vi "Dielectric vs Temperature - freq (4192A) Delay - Copy.vi"() -> ()   [LabVIEW 2013]
uses:
  <vilib>/Instr/_visa.llb/VISA Configure Serial Port (Instr).vi
  <vilib>/Utility/file.llb/Write To Spreadsheet File (DBL).vi
  Instance           5 32Saved   K vs Temp - freq (4284A) .vi
  Instance           6 32Saved   K vs Temp - freq (4284A) .vi
  Instance          15 32Saved   K vs Temp - freq (4284A) .vi
  Instance          16 32Saved   K vs Temp - freq (4284A) .vi
  Instance           7 32Saved   K vs Temp - freq (4284A) .vi
  Instance           8 32Saved   K vs Temp - freq (4284A) .vi
  Instance           9 32Saved   K vs Temp - freq (4284A) .vi
  Instance          10 32Saved   K vs Temp - freq (4284A) .vi
  Instance          11 32Saved   K vs Temp - freq (4284A) .vi
  Instance          12 32Saved   K vs Temp - freq (4284A) .vi
  Instance          13 32Saved   K vs Temp - freq (4284A) .vi
  Instance          14 32Saved   K vs Temp - freq (4284A) .vi
  Instance          17 32Saved   K vs Temp - freq (4284A) .vi
  Instance          18 32Saved   K vs Temp - freq (4284A) .vi
  Instance          19 32Saved   K vs Temp - freq (4284A) .vi
  Instance          20 32Saved   K vs Temp - freq (4284A) .vi
  Instance          21 32Saved   K vs Temp - freq (4284A) .vi
  Instance          22 32Saved   K vs Temp - freq (4284A) .vi
  Instance          23 32Saved   K vs Temp - freq (4284A) .vi
  Instance          25 32Saved   K vs Temp - freq (4284A) .vi
  Instance          24 32Saved   K vs Temp - freq (4284A) .vi
  Instance          26 32Saved   K vs Temp - freq (4284A) .vi
panel:
  in  "Freq Value (Hz) (1MHz)":dbl=1000000.0
  out "tand1M":dbl
  out "K1M":dbl
  out "C1M":dbl
  out "Temp1MHz":dbl format="%#_3g"
  in  "Freq Value (Hz) (500kHz)":dbl=500000.0
  out "tand500k":dbl
  out "K500k":dbl
  out "C500k":dbl
  out "Temp500kHz":dbl format="%#_3g"
  in  "Freq Value (Hz) (250kHz)":dbl=250000.0
  out "tand250k":dbl
  out "K250k":dbl
  out "C250k":dbl
  out "Temp250kHz":dbl format="%#_3g"
  in  "Freq Value (Hz) (100kHz)":dbl=100000.0
  out "tand100k":dbl
  out "K100k":dbl
  out "C100k":dbl
  out "Temp100kHz":dbl format="%#_3g"
  in  "Freq Value (Hz) (50kHz)":dbl=50000.0
  out "tand50k":dbl
  out "K50k":dbl
  out "C50k":dbl
  out "Temp50kHz":dbl format="%#_3g"
  in  "Freq Value (Hz) (25kHz)":dbl=25000.0
  out "tand25k":dbl
  out "K25k":dbl
  out "C25k":dbl
  out "Temp25kHz":dbl format="%#_3g"
  in  "Freq Value (Hz) (10kHz)":dbl=10000.0
  out "tand10k":dbl
  out "K10k":dbl
  out "C10k":dbl
  out "Temp10kHz":dbl format="%#_3g"
  in  "Freq Value (Hz) (5kHz)":dbl=5000.0
  out "tand5k":dbl
  out "K5k":dbl
  out "C5k":dbl
  out "Temp5kHz":dbl format="%#_3g"
  in  "Freq Value (Hz) (2.5kHz)":dbl=2500.0
  out "tand2.5k":dbl
  out "K2.5k":dbl
  out "C2.5k":dbl
  out "Temp2.5kHz":dbl format="%#_3g"
  in  "Freq Value (Hz) (1kHz)":dbl=1000.0
  out "tand1k":dbl
  out "K1k":dbl
  out "C1k":dbl
  out "Temp1kHz":dbl format="%#_3g"
  in  "tand500k":dbl[](array[numeric])
  in  "K500k":dbl[](array[numeric])
  in  "Temp500k":dbl[](array[numeric])
  out "Temp500Hz":dbl format="%#_3g"
  out "C500":dbl
  out "?":dbl
  out "tand500":dbl
  in  "Freq Value (Hz) (500Hz)":dbl=500.0
  in  "Freq Value (Hz) (250Hz)":dbl=250.0
  in  "Freq Value (Hz) (100Hz)":dbl=100.0
  in  "Freq Value (Hz) (50Hz)":dbl=50.0
  in  "Freq Value (Hz) (25Hz)":dbl=25.0
  in  "tand100k":dbl[](array[numeric])
  in  "tand10k":dbl[](array[numeric])
  in  "tand1k":dbl[](array[numeric])
  in  "tand100":dbl[](array[numeric])
  in  "K100k":dbl[](array[numeric])
  in  "K10k":dbl[](array[numeric])
  in  "K1k":dbl[](array[numeric])
  in  "K100":dbl[](array[numeric])
  in  "Temp100k":dbl[](array[numeric])
  in  "Temp10k":dbl[](array[numeric])
  in  "Temp1k":dbl[](array[numeric])
  in  "Temp100":dbl[](array[numeric])
  out "Temp250Hz":dbl format="%#_3g"
  out "Temp100Hz":dbl format="%#_3g"
  out "tand25":dbl
  out "Temp50Hz":dbl format="%#_3g"
  in  "Start":bool
  out "Thickness":dbl
  out "Area":dbl
  in  "stop":bool
  out "tand250":dbl
  out "tand100":dbl
  out "tand50":dbl
  out "K250":dbl
  out "K100":dbl
  out "K50":dbl
  out "K25":dbl
  out "C250":dbl
  out "C100":dbl
  out "C50":dbl
  out "C25":dbl
  out "Temp25Hz":dbl format="%#_3g"
  out "Dielectric Loss vs. Temperature":cluster{"Y":dbl[], "Y":dbl[]}[](graph)
  out "Relative Permittivity vs. Temperature":cluster{"Y":dbl[], "Y":dbl[]}[](graph)
  in  "Comment (Sample's Name, compositions, whatever you want,..)":string
  in  "Thickness (mm)":dbl
  in  "Diameter (mm)":dbl
  in  "Path & File Name (*.txt)":path
  # "Temperature (C)"
  # "Frequency (Hz)"
  # "Capacitance (F)"
  # "Relative Permittivity"
  # "Dielectric Loss"
  # "Sample Details"
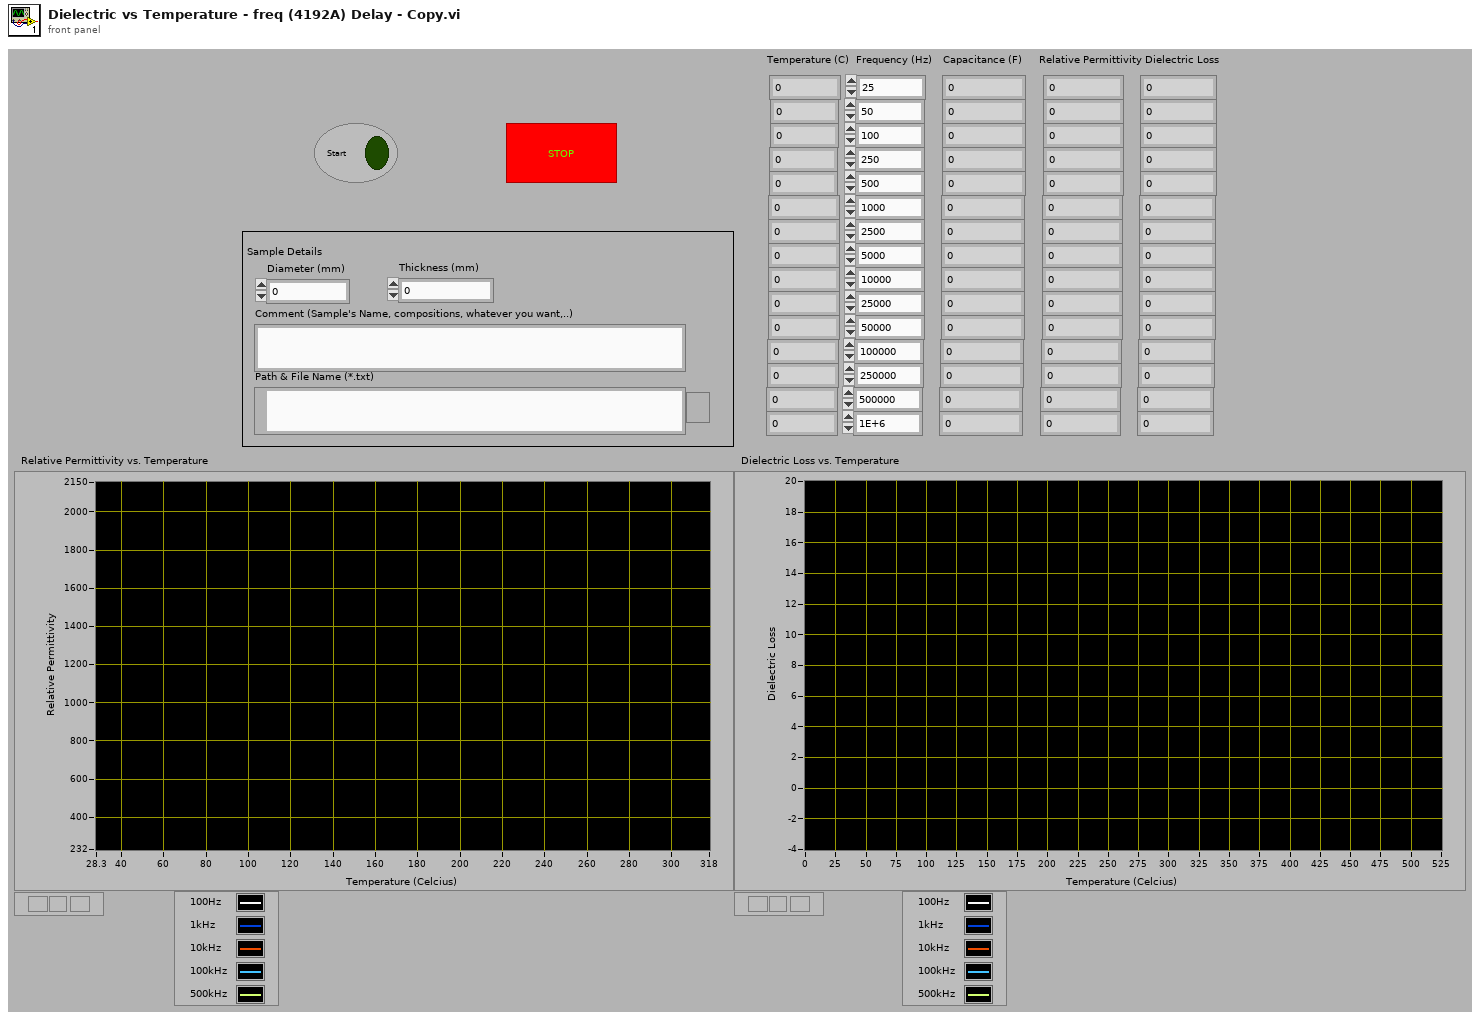
[diagram p1: front panel]
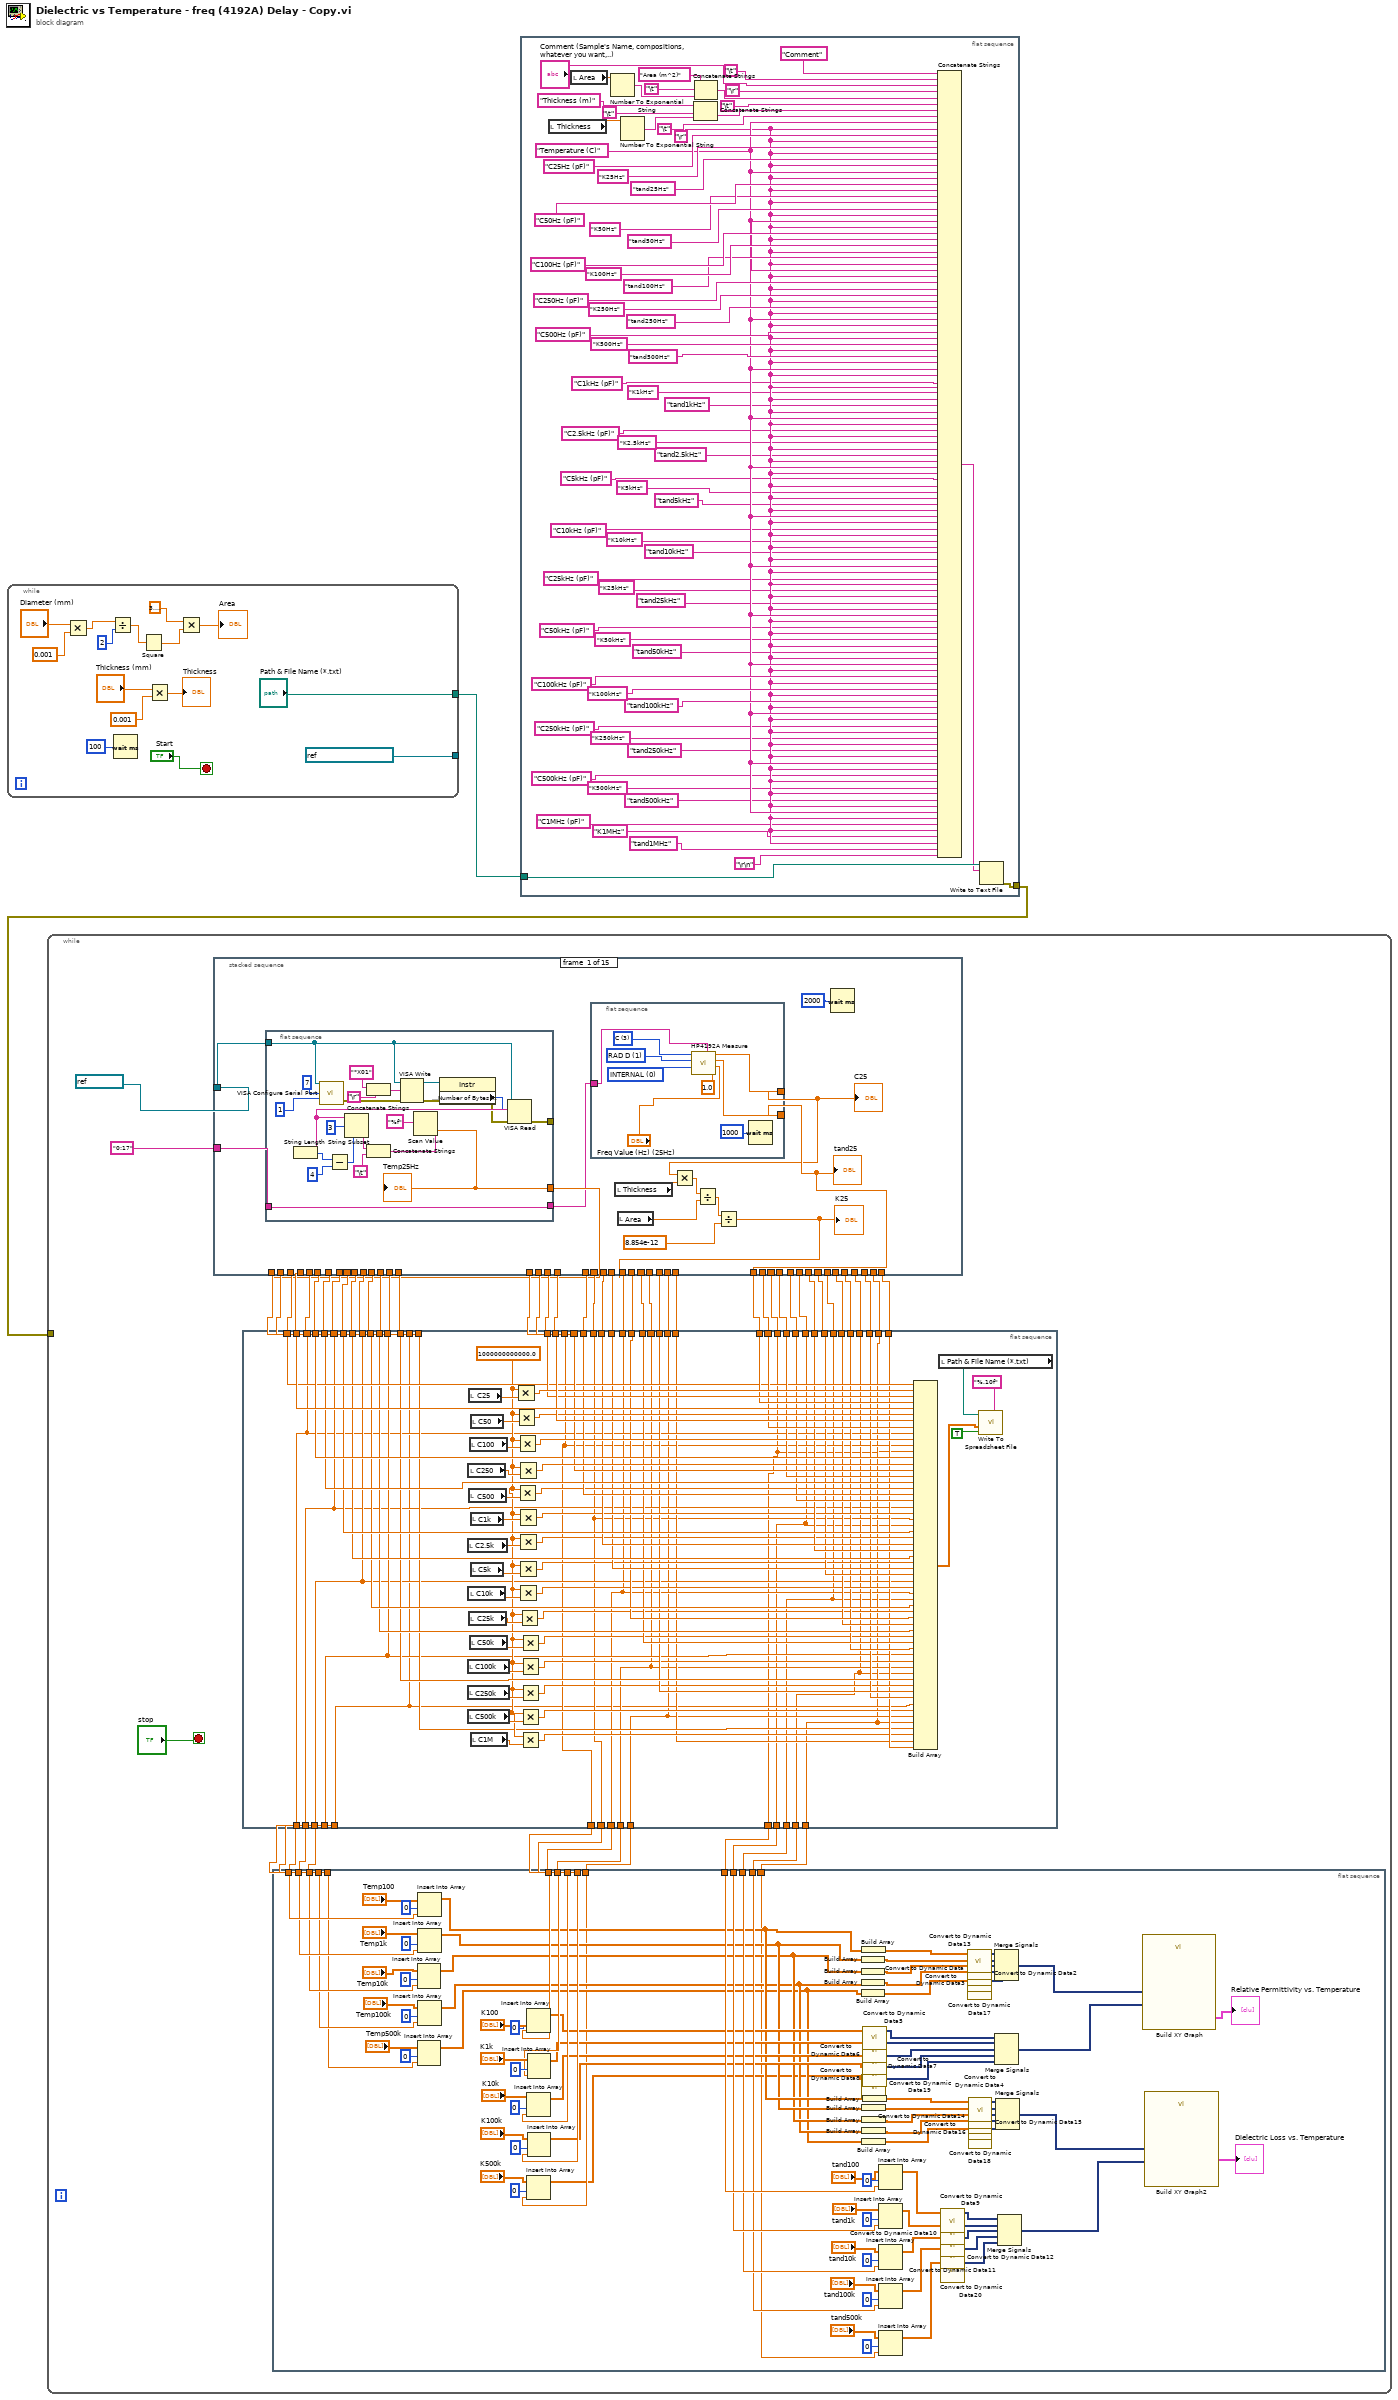
[diagram p0: block diagram]
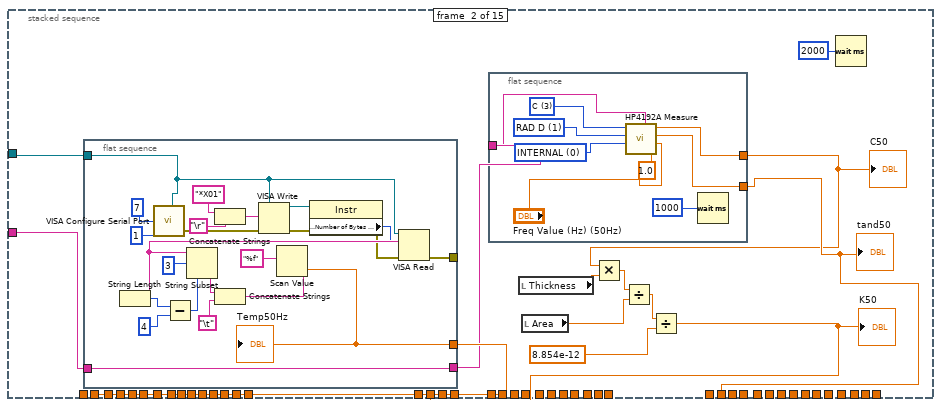
[diagram p2: hidden frame]
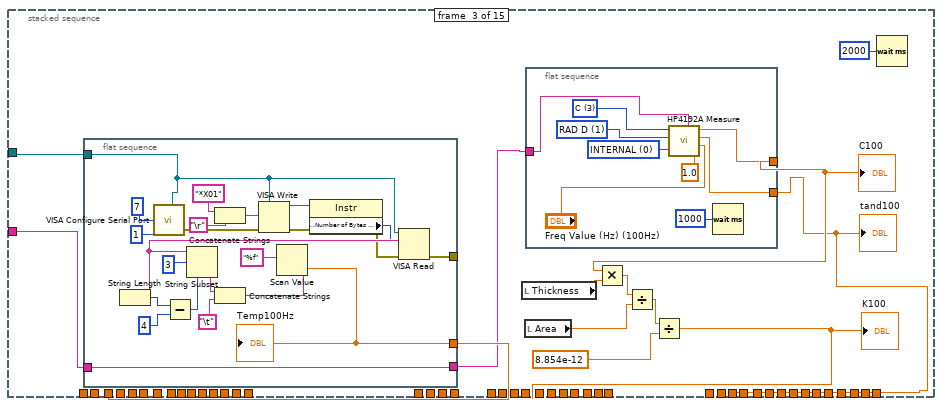
[diagram p3: hidden frame]
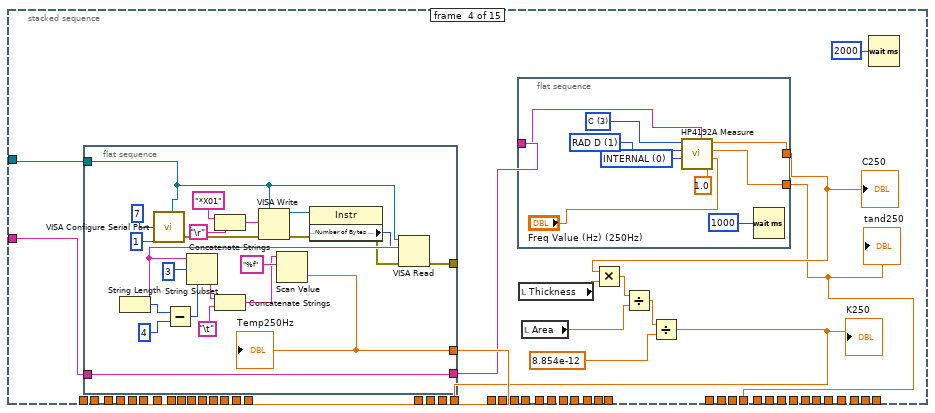
[diagram p4: hidden frame]
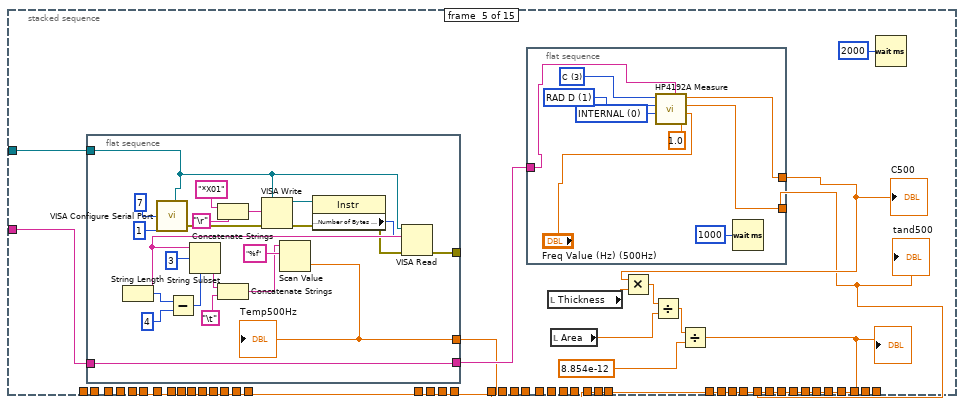
[diagram p5: hidden frame]
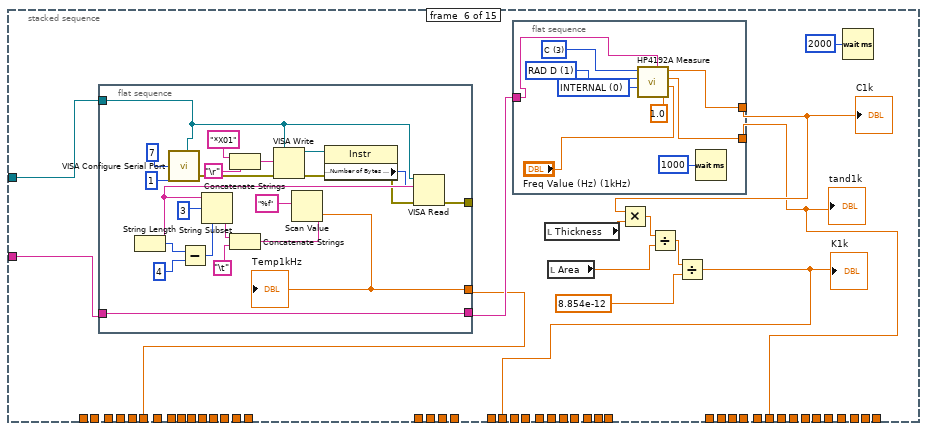
[diagram p6: hidden frame]
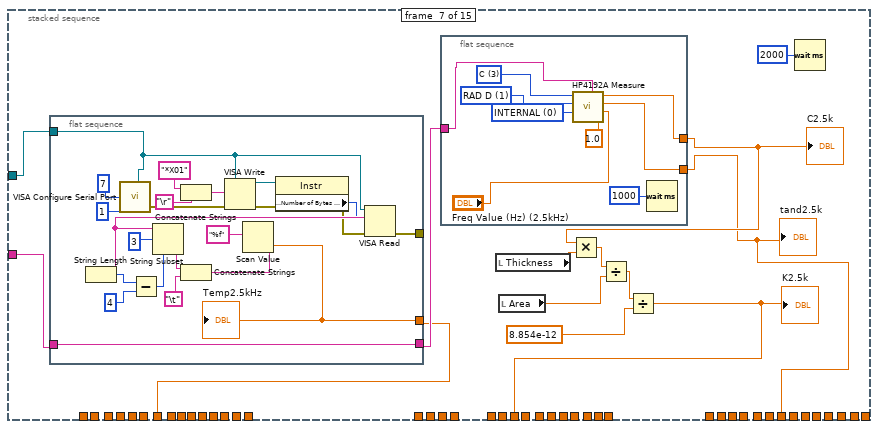
[diagram p7: hidden frame]
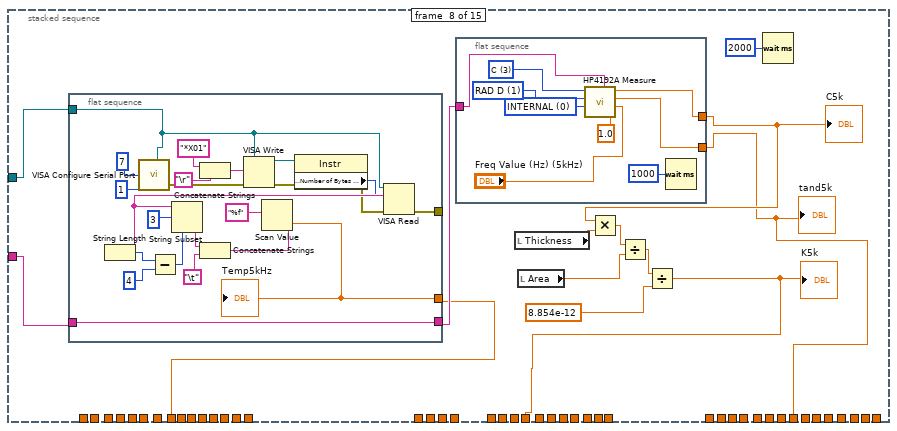
[diagram p8: hidden frame]
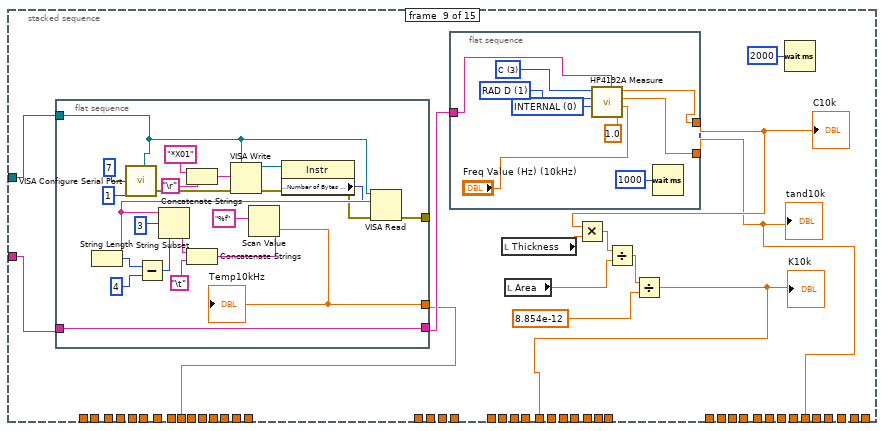
[diagram p9: hidden frame]
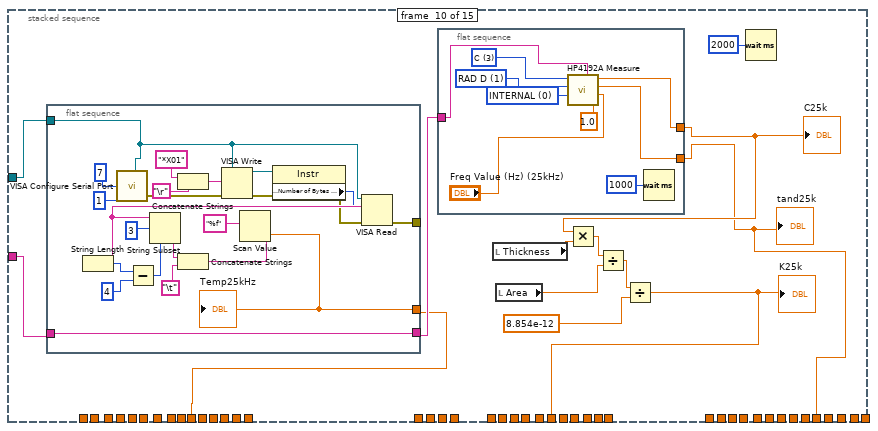
[diagram p10: hidden frame]
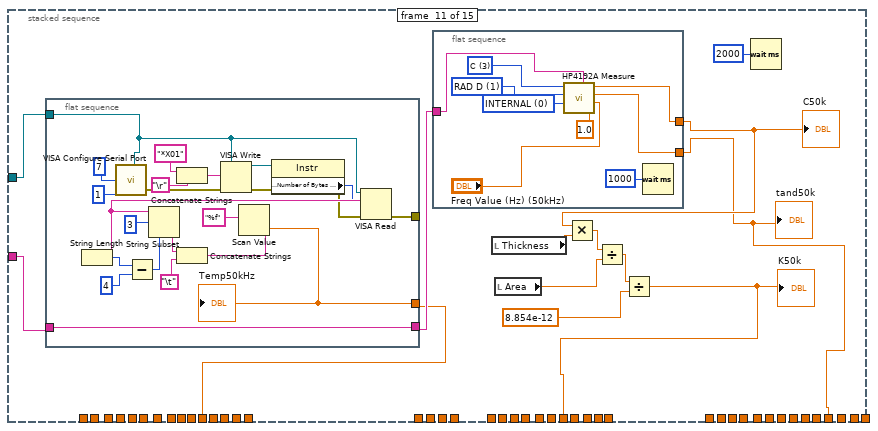
[diagram p11: hidden frame]
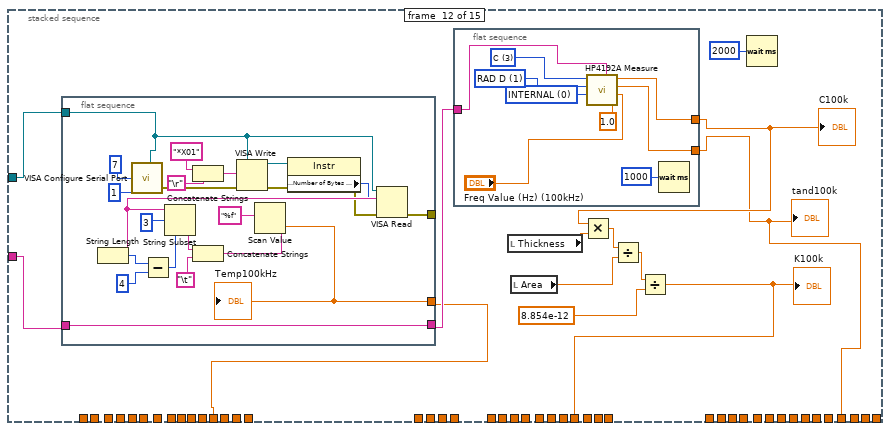
[diagram p12: hidden frame]
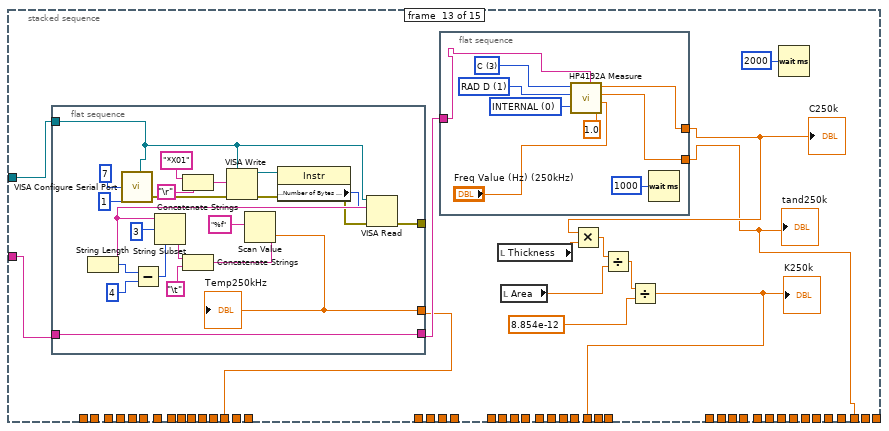
[diagram p13: hidden frame]
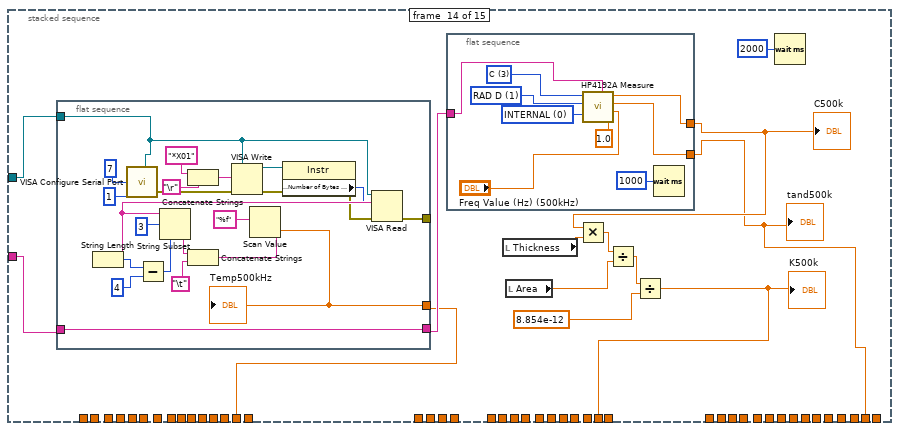
[diagram p14: hidden frame]
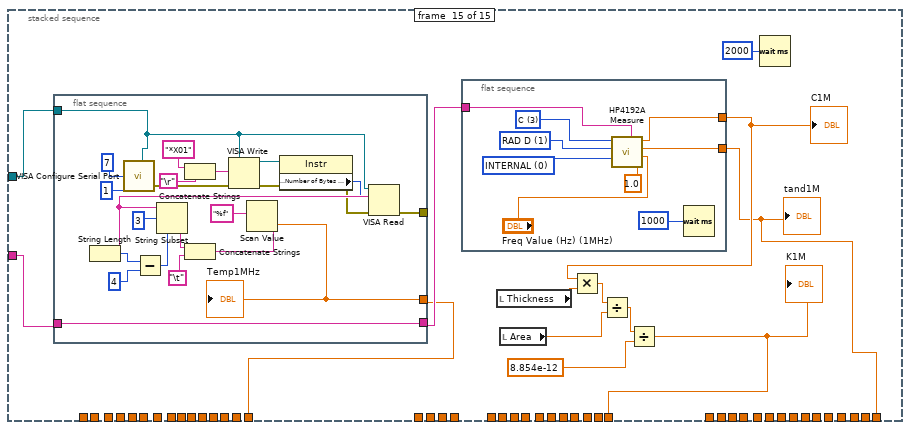
[diagram p15: hidden frame]
diagram:
  n1 = while {
    tunnel: ["Path & File Name (*.txt)"] -> w2
    tunnel: [refnum<visa-resource-name> "GPIB0::17::INSTR" ("VISA Omega (Serial - COM1)")] -> _
    stop <- "Start" stop-if-true
    n2 = Multiply(x="Diameter (mm)", y=0.001) -> (x*y=w12:dbl)
    n3 = Divide(x=w12, y=2) -> (x/y=w7:dbl)
    n4 = Wait (ms)(milliseconds to wait=u32 100) -> ()  [unwired: 1 out]
    n5 = Square(x=w7) -> (x^2=w8:dbl)
    n6 = Multiply(x="Thickness (mm)", y=0.001) -> (x*y=→"Thickness":dbl)
    n7 = Multiply(x=3.141592653589793, y=w8) -> (x*y=→"Area":dbl)
  }
  n8 = while {
    tunnel: w1 -> [_]
    stop <- "stop" stop-if-true
    n9 = stacked-sequence {
      tunnel: refnum<visa-resource-name> "COM1" ("VISA Omega (Serial - COM1)") -> [w269 w314 w359 w404 w442 w487 w532 w577 w622 w667 w712 w757 w802 w847 w892]
      tunnel: "0:17" -> [w268 w313 w358 w403 w443 w486 w531 w576 w621 w666 w711 w756 w801 w846 w891]
      tunnel: [w262 _ _ _ _ _ _ _ _ _ _ _ _ _ _] -> w68
      tunnel: [_ w307 _ _ _ _ _ _ _ _ _ _ _ _ _] -> w79
      tunnel: [_ _ w352 _ _ _ _ _ _ _ _ _ _ _ _] -> w78
      tunnel: [_ _ _ w397 _ _ _ _ _ _ _ _ _ _ _] -> w77
      tunnel: [w261 _ _ _ _ _ _ _ _ _ _ _ _ _ _] -> w76
      tunnel: [_ w306 _ _ _ _ _ _ _ _ _ _ _ _ _] -> w75
      tunnel: [_ _ w351 _ _ _ _ _ _ _ _ _ _ _ _] -> w74
      tunnel: [_ _ _ w396 _ _ _ _ _ _ _ _ _ _ _] -> w73
      tunnel: [w259 _ _ _ _ _ _ _ _ _ _ _ _ _ _] -> w72
      tunnel: [_ w305 _ _ _ _ _ _ _ _ _ _ _ _ _] -> w71
      tunnel: [_ _ w349 _ _ _ _ _ _ _ _ _ _ _ _] -> w70
      tunnel: [_ _ _ w393 _ _ _ _ _ _ _ _ _ _ _] -> w69
      tunnel: [_ _ _ _ w440 _ _ _ _ _ _ _ _ _ _] -> w67
      tunnel: [_ _ _ _ w439 _ _ _ _ _ _ _ _ _ _] -> w66
      tunnel: [_ _ _ _ w438 _ _ _ _ _ _ _ _ _ _] -> w65
      tunnel: [_ _ _ _ _ w485 _ _ _ _ _ _ _ _ _] -> w64
      tunnel: [_ _ _ _ _ w484 _ _ _ _ _ _ _ _ _] -> w63
      tunnel: [_ _ _ _ _ w483 _ _ _ _ _ _ _ _ _] -> w62
      tunnel: [_ _ _ _ _ _ w530 _ _ _ _ _ _ _ _] -> w61
      tunnel: [_ _ _ _ _ _ w529 _ _ _ _ _ _ _ _] -> w60
      tunnel: [_ _ _ _ _ _ w528 _ _ _ _ _ _ _ _] -> w59
      tunnel: [_ _ _ _ _ _ _ w575 _ _ _ _ _ _ _] -> w58
      tunnel: [_ _ _ _ _ _ _ w574 _ _ _ _ _ _ _] -> w57
      tunnel: [_ _ _ _ _ _ _ w573 _ _ _ _ _ _ _] -> w56
      tunnel: [_ _ _ _ _ _ _ _ w620 _ _ _ _ _ _] -> w55
      tunnel: [_ _ _ _ _ _ _ _ w619 _ _ _ _ _ _] -> w54
      tunnel: [_ _ _ _ _ _ _ _ w618 _ _ _ _ _ _] -> w53
      tunnel: [_ _ _ _ _ _ _ _ _ w665 _ _ _ _ _] -> w52
      tunnel: [_ _ _ _ _ _ _ _ _ w664 _ _ _ _ _] -> w51
      tunnel: [_ _ _ _ _ _ _ _ _ w663 _ _ _ _ _] -> w50
      tunnel: [_ _ _ _ _ _ _ _ _ _ w710 _ _ _ _] -> w49
      tunnel: [_ _ _ _ _ _ _ _ _ _ w709 _ _ _ _] -> w48
      tunnel: [_ _ _ _ _ _ _ _ _ _ w708 _ _ _ _] -> w47
      tunnel: [_ _ _ _ _ _ _ _ _ _ _ w755 _ _ _] -> w46
      tunnel: [_ _ _ _ _ _ _ _ _ _ _ w754 _ _ _] -> w45
      tunnel: [_ _ _ _ _ _ _ _ _ _ _ w753 _ _ _] -> w44
      tunnel: [_ _ _ _ _ _ _ _ _ _ _ _ w800 _ _] -> w43
      tunnel: [_ _ _ _ _ _ _ _ _ _ _ _ w799 _ _] -> w42
      tunnel: [_ _ _ _ _ _ _ _ _ _ _ _ w798 _ _] -> w41
      tunnel: [_ _ _ _ _ _ _ _ _ _ _ _ _ w845 _] -> w40
      tunnel: [_ _ _ _ _ _ _ _ _ _ _ _ _ w844 _] -> w39
      tunnel: [_ _ _ _ _ _ _ _ _ _ _ _ _ w843 _] -> w38
      tunnel: [_ _ _ _ _ _ _ _ _ _ _ _ _ _ w890] -> w35
      tunnel: [_ _ _ _ _ _ _ _ _ _ _ _ _ _ w889] -> w36
      tunnel: [_ _ _ _ _ _ _ _ _ _ _ _ _ _ w888] -> w37
      frame #0 {
        n10 = flat-sequence {
          tunnel: w269 -> [w282]
          tunnel: [w281] -> _
          tunnel: [w280] -> w262
          tunnel: w268 -> [w279]
          tunnel: [w279] -> w260
          frame #0 {
            n11 = call-poly "VISA Configure Serial Port"("VISA resource name"=w282, "data bits (8)"=7, "parity (0:none)"=1) -> ("error out"=w287:errorcluster)  [unwired: 11 in, 1 out]
            n12 = Concatenate Strings("*X01", "\r") -> (w290:string)
            n13 = VISA Write(VISA resource name=w282, write buffer=w290, error in (no error)=w287) -> (VISA resource name out=w301:refnum<visa-resource-name>, error out=w291:errorcluster)  [unwired: 1 out]
            n14 = property class="Instr"(reference=w301, error in=w291) -> (error out=w292:errorcluster, "Serial Settings:Number of Bytes at Serial Port"=w293:u32)  [unwired: 1 out]
            n15 = VISA Read(VISA resource name=w282, byte count=w293, error in (no error)=w292) -> (read buffer=w294:string, error out=w281:errorcluster)  [unwired: 2 out]
            n16 = String Length(string=w294) -> (length=w296:i32)
            n17 = Subtract(x=w296, y=4) -> (x-y=w298:i32)
            n18 = String Subset(string=w294, offset (0)=3, length (rest)=w298) -> (substring=w299:string)
            n19 = Concatenate Strings(w299, "\t") -> (w283:string)
            n20 = Scan Value(string=w283, format string="%f") -> (value=w280:dbl)  [unwired: 1 in, 1 out]
            "Temp25Hz" <- w280
          }
        }
        n21 = flat-sequence {
          tunnel: w260 -> [w276]
          tunnel: [w274] -> w259
          tunnel: [w275] -> w258
          frame #0 {
            w271 = i16 1 items=["DEG Q", "RAD D", "         R/G"] ("function B (deg q:0)")
            w272 = i16 3 items=["Z/Y", "R/G", "L", "C"] ("function A (z/y:0)")
            w273 = i16 0 items=["INTERNAL", "EXTERNAL", "HOLD/MANUAL"] ("trigger (internal:0)")
            n22 = call "HP4192A Measure.vi"("OSC level (V)"=1.0, "test signal\nfreq (Hz)"="Freq Value (Hz) (25Hz)", "GPIB addess"=w276, "trigger (internal:0)"=w273, "function B (deg q:0)"=w271, "function A (z/y:0)"=w272) -> ("display B"=w274:dbl, "display A"=w275:dbl)  [unwired: 4 in]
            n23 = Wait (ms)(milliseconds to wait=u32 1000) -> ()  [unwired: 1 out]
          }
        }
        n24 = local read "Thickness"() -> (w267:dbl)
        n25 = local read "Area"() -> (w265:dbl)
        n26 = Multiply(x=w258, y=w267) -> (x*y=w266:dbl)
        n27 = Divide(x=w266, y=w265) -> (x/y=w264:dbl)
        n28 = Divide(x=w264, y=8.854e-12) -> (x/y=w261:dbl)
        "K25" <- w261
        n29 = Wait (ms)(milliseconds to wait=u32 2000) -> ()  [unwired: 1 out]
        "C25" <- w258
        "tand25" <- w259
      }
      frame #1 {
        n30 = flat-sequence {
          tunnel: w314 -> [w327]
          tunnel: [w326] -> _
          tunnel: [w325] -> w307
          tunnel: w313 -> [w324]
          tunnel: [w324] -> w303
          frame #0 {
            n31 = call-poly "VISA Configure Serial Port"("VISA resource name"=w327, "data bits (8)"=7, "parity (0:none)"=1) -> ("error out"=w332:errorcluster)  [unwired: 11 in, 1 out]
            n32 = Concatenate Strings("*X01", "\r") -> (w335:string)
            n33 = VISA Write(VISA resource name=w327, write buffer=w335, error in (no error)=w332) -> (VISA resource name out=w346:refnum<visa-resource-name>, error out=w336:errorcluster)  [unwired: 1 out]
            n34 = property class="Instr"(reference=w346, error in=w336) -> (error out=w337:errorcluster, "Serial Settings:Number of Bytes at Serial Port"=w338:u32)  [unwired: 1 out]
            n35 = VISA Read(VISA resource name=w327, byte count=w338, error in (no error)=w337) -> (read buffer=w339:string, error out=w326:errorcluster)  [unwired: 2 out]
            n36 = String Length(string=w339) -> (length=w341:i32)
            n37 = Subtract(x=w341, y=4) -> (x-y=w343:i32)
            n38 = String Subset(string=w339, offset (0)=3, length (rest)=w343) -> (substring=w344:string)
            n39 = Concatenate Strings(w344, "\t") -> (w328:string)
            n40 = Scan Value(string=w328, format string="%f") -> (value=w325:dbl)  [unwired: 1 in, 1 out]
            "Temp50Hz" <- w325
          }
        }
        n41 = flat-sequence {
          tunnel: w303 -> [w318]
          tunnel: [w316] -> w305
          tunnel: [w317] -> w304
          frame #0 {
            w315 = i16 0 items=["INTERNAL", "EXTERNAL", "HOLD/MANUAL"] ("trigger (internal:0)")
            w321 = i16 1 items=["DEG Q", "RAD D", "         R/G"] ("function B (deg q:0)")
            w322 = i16 3 items=["Z/Y", "R/G", "L", "C"] ("function A (z/y:0)")
            n42 = call "HP4192A Measure.vi"("OSC level (V)"=1.0, "test signal\nfreq (Hz)"="Freq Value (Hz) (50Hz)", "GPIB addess"=w318, "trigger (internal:0)"=w315, "function B (deg q:0)"=w321, "function A (z/y:0)"=w322) -> ("display B"=w316:dbl, "display A"=w317:dbl)  [unwired: 4 in]
            n43 = Wait (ms)(milliseconds to wait=u32 1000) -> ()  [unwired: 1 out]
          }
        }
        n44 = local read "Thickness"() -> (w312:dbl)
        n45 = local read "Area"() -> (w310:dbl)
        n46 = Multiply(x=w304, y=w312) -> (x*y=w311:dbl)
        n47 = Divide(x=w311, y=w310) -> (x/y=w309:dbl)
        n48 = Divide(x=w309, y=8.854e-12) -> (x/y=w306:dbl)
        "K50" <- w306
        n49 = Wait (ms)(milliseconds to wait=u32 2000) -> ()  [unwired: 1 out]
        "tand50" <- w305
        "C50" <- w304
      }
      frame #2 {
        n50 = flat-sequence {
          tunnel: w359 -> [w372]
          tunnel: [w371] -> _
          tunnel: [w370] -> w352
          tunnel: w358 -> [w369]
          tunnel: [w369] -> w348
          frame #0 {
            n51 = call-poly "VISA Configure Serial Port"("VISA resource name"=w372, "data bits (8)"=7, "parity (0:none)"=1) -> ("error out"=w377:errorcluster)  [unwired: 11 in, 1 out]
            n52 = Concatenate Strings("*X01", "\r") -> (w380:string)
            n53 = VISA Write(VISA resource name=w372, write buffer=w380, error in (no error)=w377) -> (VISA resource name out=w391:refnum<visa-resource-name>, error out=w381:errorcluster)  [unwired: 1 out]
            n54 = property class="Instr"(reference=w391, error in=w381) -> (error out=w382:errorcluster, "Serial Settings:Number of Bytes at Serial Port"=w383:u32)  [unwired: 1 out]
            n55 = VISA Read(VISA resource name=w372, byte count=w383, error in (no error)=w382) -> (read buffer=w384:string, error out=w371:errorcluster)  [unwired: 2 out]
            n56 = String Length(string=w384) -> (length=w386:i32)
            n57 = Subtract(x=w386, y=4) -> (x-y=w388:i32)
            n58 = String Subset(string=w384, offset (0)=3, length (rest)=w388) -> (substring=w389:string)
            n59 = Concatenate Strings(w389, "\t") -> (w373:string)
            n60 = Scan Value(string=w373, format string="%f") -> (value=w370:dbl)  [unwired: 1 in, 1 out]
            "Temp100Hz" <- w370
          }
        }
        n61 = local read "Thickness"() -> (w357:dbl)
        n62 = local read "Area"() -> (w355:dbl)
        n63 = flat-sequence {
          tunnel: w348 -> [w363]
          tunnel: [w361] -> w349
          tunnel: [w362] -> w350
          frame #0 {
            w360 = i16 0 items=["INTERNAL", "EXTERNAL", "HOLD/MANUAL"] ("trigger (internal:0)")
            w366 = i16 1 items=["DEG Q", "RAD D", "         R/G"] ("function B (deg q:0)")
            w367 = i16 3 items=["Z/Y", "R/G", "L", "C"] ("function A (z/y:0)")
            n64 = call "HP4192A Measure.vi"("OSC level (V)"=1.0, "test signal\nfreq (Hz)"="Freq Value (Hz) (100Hz)", "GPIB addess"=w363, "trigger (internal:0)"=w360, "function B (deg q:0)"=w366, "function A (z/y:0)"=w367) -> ("display B"=w361:dbl, "display A"=w362:dbl)  [unwired: 4 in]
            n65 = Wait (ms)(milliseconds to wait=u32 1000) -> ()  [unwired: 1 out]
          }
        }
        n66 = Multiply(x=w350, y=w357) -> (x*y=w356:dbl)
        n67 = Divide(x=w356, y=w355) -> (x/y=w354:dbl)
        n68 = Divide(x=w354, y=8.854e-12) -> (x/y=w351:dbl)
        "K100" <- w351
        n69 = Wait (ms)(milliseconds to wait=u32 2000) -> ()  [unwired: 1 out]
        "C100" <- w350
        "tand100" <- w349
      }
      frame #3 {
        n70 = flat-sequence {
          tunnel: w404 -> [w417]
          tunnel: [w416] -> _
          tunnel: [w415] -> w397
          tunnel: w403 -> [w414]
          tunnel: [w414] -> w395
          frame #0 {
            n71 = call-poly "VISA Configure Serial Port"("VISA resource name"=w417, "data bits (8)"=7, "parity (0:none)"=1) -> ("error out"=w422:errorcluster)  [unwired: 11 in, 1 out]
            n72 = Concatenate Strings("*X01", "\r") -> (w425:string)
            n73 = VISA Write(VISA resource name=w417, write buffer=w425, error in (no error)=w422) -> (VISA resource name out=w436:refnum<visa-resource-name>, error out=w426:errorcluster)  [unwired: 1 out]
            n74 = property class="Instr"(reference=w436, error in=w426) -> (error out=w427:errorcluster, "Serial Settings:Number of Bytes at Serial Port"=w428:u32)  [unwired: 1 out]
            n75 = VISA Read(VISA resource name=w417, byte count=w428, error in (no error)=w427) -> (read buffer=w429:string, error out=w416:errorcluster)  [unwired: 2 out]
            n76 = String Length(string=w429) -> (length=w431:i32)
            n77 = Subtract(x=w431, y=4) -> (x-y=w433:i32)
            n78 = String Subset(string=w429, offset (0)=3, length (rest)=w433) -> (substring=w434:string)
            n79 = Concatenate Strings(w434, "\t") -> (w418:string)
            n80 = Scan Value(string=w418, format string="%f") -> (value=w415:dbl)  [unwired: 1 in, 1 out]
            "Temp250Hz" <- w415
          }
        }
        n81 = flat-sequence {
          tunnel: w395 -> [w408]
          tunnel: [w406] -> w393
          tunnel: [w407] -> w394
          frame #0 {
            w405 = i16 0 items=["INTERNAL", "EXTERNAL", "HOLD/MANUAL"] ("trigger (internal:0)")
            w411 = i16 1 items=["DEG Q", "RAD D", "         R/G"] ("function B (deg q:0)")
            w412 = i16 3 items=["Z/Y", "R/G", "L", "C"] ("function A (z/y:0)")
            n82 = call "HP4192A Measure.vi"("OSC level (V)"=1.0, "test signal\nfreq (Hz)"="Freq Value (Hz) (250Hz)", "GPIB addess"=w408, "trigger (internal:0)"=w405, "function B (deg q:0)"=w411, "function A (z/y:0)"=w412) -> ("display B"=w406:dbl, "display A"=w407:dbl)  [unwired: 4 in]
            n83 = Wait (ms)(milliseconds to wait=u32 1000) -> ()  [unwired: 1 out]
          }
        }
        n84 = local read "Thickness"() -> (w402:dbl)
        n85 = local read "Area"() -> (w400:dbl)
        n86 = Multiply(x=w394, y=w402) -> (x*y=w401:dbl)
        n87 = Divide(x=w401, y=w400) -> (x/y=w399:dbl)
        n88 = Divide(x=w399, y=8.854e-12) -> (x/y=w396:dbl)
        "K250" <- w396
        n89 = Wait (ms)(milliseconds to wait=u32 2000) -> ()  [unwired: 1 out]
        "C250" <- w394
        "tand250" <- w393
      }
      frame #4 {
        n90 = flat-sequence {
          tunnel: w442 -> [w462]
          tunnel: [w461] -> _
          tunnel: [w460] -> w440
          tunnel: w443 -> [w459]
          tunnel: [w459] -> w441
          frame #0 {
            n91 = call-poly "VISA Configure Serial Port"("VISA resource name"=w462, "data bits (8)"=7, "parity (0:none)"=1) -> ("error out"=w467:errorcluster)  [unwired: 11 in, 1 out]
            n92 = Concatenate Strings("*X01", "\r") -> (w470:string)
            n93 = VISA Write(VISA resource name=w462, write buffer=w470, error in (no error)=w467) -> (VISA resource name out=w481:refnum<visa-resource-name>, error out=w471:errorcluster)  [unwired: 1 out]
            n94 = property class="Instr"(reference=w481, error in=w471) -> (error out=w472:errorcluster, "Serial Settings:Number of Bytes at Serial Port"=w473:u32)  [unwired: 1 out]
            n95 = VISA Read(VISA resource name=w462, byte count=w473, error in (no error)=w472) -> (read buffer=w474:string, error out=w461:errorcluster)  [unwired: 2 out]
            n96 = String Length(string=w474) -> (length=w476:i32)
            n97 = Subtract(x=w476, y=4) -> (x-y=w478:i32)
            n98 = String Subset(string=w474, offset (0)=3, length (rest)=w478) -> (substring=w479:string)
            n99 = Concatenate Strings(w479, "\t") -> (w463:string)
            n100 = Scan Value(string=w463, format string="%f") -> (value=w460:dbl)  [unwired: 1 in, 1 out]
            "Temp500Hz" <- w460
          }
        }
        n101 = flat-sequence {
          tunnel: w441 -> [w451]
          tunnel: [w453] -> w438
          tunnel: [w452] -> w444
          frame #0 {
            w450 = i16 0 items=["INTERNAL", "EXTERNAL", "HOLD/MANUAL"] ("trigger (internal:0)")
            w456 = i16 1 items=["DEG Q", "RAD D", "         R/G"] ("function B (deg q:0)")
            w457 = i16 3 items=["Z/Y", "R/G", "L", "C"] ("function A (z/y:0)")
            n102 = call "HP4192A Measure.vi"("OSC level (V)"=1.0, "test signal\nfreq (Hz)"="Freq Value (Hz) (500Hz)", "GPIB addess"=w451, "trigger (internal:0)"=w450, "function B (deg q:0)"=w456, "function A (z/y:0)"=w457) -> ("display B"=w453:dbl, "display A"=w452:dbl)  [unwired: 4 in]
            n103 = Wait (ms)(milliseconds to wait=u32 1000) -> ()  [unwired: 1 out]
          }
        }
        n104 = local read "Thickness"() -> (w449:dbl)
        n105 = local read "Area"() -> (w447:dbl)
        n106 = Multiply(x=w444, y=w449) -> (x*y=w448:dbl)
        n107 = Divide(x=w448, y=w447) -> (x/y=w446:dbl)
        n108 = Divide(x=w446, y=8.854e-12) -> (x/y=w439:dbl)
        "?" <- w439
        n109 = Wait (ms)(milliseconds to wait=u32 2000) -> ()  [unwired: 1 out]
        "C500" <- w444
        "tand500" <- w438
      }
      frame #5 {
        n110 = flat-sequence {
          tunnel: w487 -> [w507]
          tunnel: [w506] -> _
          tunnel: [w505] -> w485
          tunnel: w486 -> [w504]
          tunnel: [w504] -> w489
          frame #0 {
            n111 = call-poly "VISA Configure Serial Port"("VISA resource name"=w507, "data bits (8)"=7, "parity (0:none)"=1) -> ("error out"=w512:errorcluster)  [unwired: 11 in, 1 out]
            n112 = Concatenate Strings("*X01", "\r") -> (w515:string)
            n113 = VISA Write(VISA resource name=w507, write buffer=w515, error in (no error)=w512) -> (VISA resource name out=w526:refnum<visa-resource-name>, error out=w516:errorcluster)  [unwired: 1 out]
            n114 = property class="Instr"(reference=w526, error in=w516) -> (error out=w517:errorcluster, "Serial Settings:Number of Bytes at Serial Port"=w518:u32)  [unwired: 1 out]
            n115 = VISA Read(VISA resource name=w507, byte count=w518, error in (no error)=w517) -> (read buffer=w519:string, error out=w506:errorcluster)  [unwired: 2 out]
            n116 = String Length(string=w519) -> (length=w521:i32)
            n117 = Subtract(x=w521, y=4) -> (x-y=w523:i32)
            n118 = String Subset(string=w519, offset (0)=3, length (rest)=w523) -> (substring=w524:string)
            n119 = Concatenate Strings(w524, "\t") -> (w508:string)
            n120 = Scan Value(string=w508, format string="%f") -> (value=w505:dbl)  [unwired: 1 in, 1 out]
            "Temp1kHz" <- w505
          }
        }
        n121 = flat-sequence {
          tunnel: w489 -> [w499]
          tunnel: [w496] -> w483
          tunnel: [w497] -> w488
          frame #0 {
            w495 = i16 0 items=["INTERNAL", "EXTERNAL", "HOLD/MANUAL"] ("trigger (internal:0)")
            w501 = i16 1 items=["DEG Q", "RAD D", "         R/G"] ("function B (deg q:0)")
            w502 = i16 3 items=["Z/Y", "R/G", "L", "C"] ("function A (z/y:0)")
            n122 = call "HP4192A Measure.vi"("OSC level (V)"=1.0, "test signal\nfreq (Hz)"="Freq Value (Hz) (1kHz)", "GPIB addess"=w499, "trigger (internal:0)"=w495, "function B (deg q:0)"=w501, "function A (z/y:0)"=w502) -> ("display B"=w496:dbl, "display A"=w497:dbl)  [unwired: 4 in]
            n123 = Wait (ms)(milliseconds to wait=u32 1000) -> ()  [unwired: 1 out]
          }
        }
        n124 = local read "Thickness"() -> (w494:dbl)
        n125 = local read "Area"() -> (w492:dbl)
        n126 = Multiply(x=w488, y=w494) -> (x*y=w493:dbl)
        n127 = Divide(x=w493, y=w492) -> (x/y=w491:dbl)
        n128 = Divide(x=w491, y=8.854e-12) -> (x/y=w484:dbl)
        "K1k" <- w484
        n129 = Wait (ms)(milliseconds to wait=u32 2000) -> ()  [unwired: 1 out]
        "C1k" <- w488
        "tand1k" <- w483
      }
      frame #6 {
        n130 = flat-sequence {
          tunnel: w532 -> [w552]
          tunnel: [w551] -> _
          tunnel: [w550] -> w530
          tunnel: w531 -> [w549]
          tunnel: [w549] -> w534
          frame #0 {
            n131 = call-poly "VISA Configure Serial Port"("VISA resource name"=w552, "data bits (8)"=7, "parity (0:none)"=1) -> ("error out"=w557:errorcluster)  [unwired: 11 in, 1 out]
            n132 = Concatenate Strings("*X01", "\r") -> (w560:string)
            n133 = VISA Write(VISA resource name=w552, write buffer=w560, error in (no error)=w557) -> (VISA resource name out=w571:refnum<visa-resource-name>, error out=w561:errorcluster)  [unwired: 1 out]
            n134 = property class="Instr"(reference=w571, error in=w561) -> (error out=w562:errorcluster, "Serial Settings:Number of Bytes at Serial Port"=w563:u32)  [unwired: 1 out]
            n135 = VISA Read(VISA resource name=w552, byte count=w563, error in (no error)=w562) -> (read buffer=w564:string, error out=w551:errorcluster)  [unwired: 2 out]
            n136 = String Length(string=w564) -> (length=w566:i32)
            n137 = Subtract(x=w566, y=4) -> (x-y=w568:i32)
            n138 = String Subset(string=w564, offset (0)=3, length (rest)=w568) -> (substring=w569:string)
            n139 = Concatenate Strings(w569, "\t") -> (w553:string)
            n140 = Scan Value(string=w553, format string="%f") -> (value=w550:dbl)  [unwired: 1 in, 1 out]
            "Temp2.5kHz" <- w550
          }
        }
        n141 = flat-sequence {
          tunnel: w534 -> [w541]
          tunnel: [w543] -> w528
          tunnel: [w542] -> w533
          frame #0 {
            w540 = i16 0 items=["INTERNAL", "EXTERNAL", "HOLD/MANUAL"] ("trigger (internal:0)")
            w546 = i16 1 items=["DEG Q", "RAD D", "         R/G"] ("function B (deg q:0)")
            w547 = i16 3 items=["Z/Y", "R/G", "L", "C"] ("function A (z/y:0)")
            n142 = call "HP4192A Measure.vi"("OSC level (V)"=1.0, "test signal\nfreq (Hz)"="Freq Value (Hz) (2.5kHz)", "GPIB addess"=w541, "trigger (internal:0)"=w540, "function B (deg q:0)"=w546, "function A (z/y:0)"=w547) -> ("display B"=w543:dbl, "display A"=w542:dbl)  [unwired: 4 in]
            n143 = Wait (ms)(milliseconds to wait=u32 1000) -> ()  [unwired: 1 out]
          }
        }
        n144 = local read "Thickness"() -> (w539:dbl)
        n145 = local read "Area"() -> (w537:dbl)
        n146 = Multiply(x=w533, y=w539) -> (x*y=w538:dbl)
        n147 = Divide(x=w538, y=w537) -> (x/y=w536:dbl)
        n148 = Divide(x=w536, y=8.854e-12) -> (x/y=w529:dbl)
        "K2.5k" <- w529
        n149 = Wait (ms)(milliseconds to wait=u32 2000) -> ()  [unwired: 1 out]
        "C2.5k" <- w533
        "tand2.5k" <- w528
      }
      frame #7 {
        n150 = flat-sequence {
          tunnel: w577 -> [w597]
          tunnel: [w596] -> _
          tunnel: [w595] -> w575
          tunnel: w576 -> [w594]
          tunnel: [w594] -> w579
          frame #0 {
            n151 = call-poly "VISA Configure Serial Port"("VISA resource name"=w597, "data bits (8)"=7, "parity (0:none)"=1) -> ("error out"=w602:errorcluster)  [unwired: 11 in, 1 out]
            n152 = Concatenate Strings("*X01", "\r") -> (w605:string)
            n153 = VISA Write(VISA resource name=w597, write buffer=w605, error in (no error)=w602) -> (VISA resource name out=w616:refnum<visa-resource-name>, error out=w606:errorcluster)  [unwired: 1 out]
            n154 = property class="Instr"(reference=w616, error in=w606) -> (error out=w607:errorcluster, "Serial Settings:Number of Bytes at Serial Port"=w608:u32)  [unwired: 1 out]
            n155 = VISA Read(VISA resource name=w597, byte count=w608, error in (no error)=w607) -> (read buffer=w609:string, error out=w596:errorcluster)  [unwired: 2 out]
            n156 = String Length(string=w609) -> (length=w611:i32)
            n157 = Subtract(x=w611, y=4) -> (x-y=w613:i32)
            n158 = String Subset(string=w609, offset (0)=3, length (rest)=w613) -> (substring=w614:string)
            n159 = Concatenate Strings(w614, "\t") -> (w598:string)
            n160 = Scan Value(string=w598, format string="%f") -> (value=w595:dbl)  [unwired: 1 in, 1 out]
            "Temp5kHz" <- w595
          }
        }
        n161 = flat-sequence {
          tunnel: w579 -> [w586]
          tunnel: [w588] -> w573
          tunnel: [w587] -> w578
          frame #0 {
            w585 = i16 0 items=["INTERNAL", "EXTERNAL", "HOLD/MANUAL"] ("trigger (internal:0)")
            w591 = i16 1 items=["DEG Q", "RAD D", "         R/G"] ("function B (deg q:0)")
            w592 = i16 3 items=["Z/Y", "R/G", "L", "C"] ("function A (z/y:0)")
            n162 = call "HP4192A Measure.vi"("OSC level (V)"=1.0, "test signal\nfreq (Hz)"="Freq Value (Hz) (5kHz)", "GPIB addess"=w586, "trigger (internal:0)"=w585, "function B (deg q:0)"=w591, "function A (z/y:0)"=w592) -> ("display B"=w588:dbl, "display A"=w587:dbl)  [unwired: 4 in]
            n163 = Wait (ms)(milliseconds to wait=u32 1000) -> ()  [unwired: 1 out]
          }
        }
        n164 = local read "Thickness"() -> (w584:dbl)
        n165 = local read "Area"() -> (w582:dbl)
        n166 = Multiply(x=w578, y=w584) -> (x*y=w583:dbl)
        n167 = Divide(x=w583, y=w582) -> (x/y=w581:dbl)
        n168 = Divide(x=w581, y=8.854e-12) -> (x/y=w574:dbl)
        "K5k" <- w574
        n169 = Wait (ms)(milliseconds to wait=u32 2000) -> ()  [unwired: 1 out]
        "C5k" <- w578
        "tand5k" <- w573
      }
      frame #8 {
        n170 = flat-sequence {
          tunnel: w622 -> [w642]
          tunnel: [w641] -> _
          tunnel: [w640] -> w620
          tunnel: w621 -> [w639]
          tunnel: [w639] -> w624
          frame #0 {
            n171 = call-poly "VISA Configure Serial Port"("VISA resource name"=w642, "data bits (8)"=7, "parity (0:none)"=1) -> ("error out"=w647:errorcluster)  [unwired: 11 in, 1 out]
            n172 = Concatenate Strings("*X01", "\r") -> (w650:string)
            n173 = VISA Write(VISA resource name=w642, write buffer=w650, error in (no error)=w647) -> (VISA resource name out=w661:refnum<visa-resource-name>, error out=w651:errorcluster)  [unwired: 1 out]
            n174 = property class="Instr"(reference=w661, error in=w651) -> (error out=w652:errorcluster, "Serial Settings:Number of Bytes at Serial Port"=w653:u32)  [unwired: 1 out]
            n175 = VISA Read(VISA resource name=w642, byte count=w653, error in (no error)=w652) -> (read buffer=w654:string, error out=w641:errorcluster)  [unwired: 2 out]
            n176 = String Length(string=w654) -> (length=w656:i32)
            n177 = Subtract(x=w656, y=4) -> (x-y=w658:i32)
            n178 = String Subset(string=w654, offset (0)=3, length (rest)=w658) -> (substring=w659:string)
            n179 = Concatenate Strings(w659, "\t") -> (w643:string)
            n180 = Scan Value(string=w643, format string="%f") -> (value=w640:dbl)  [unwired: 1 in, 1 out]
            "Temp10kHz" <- w640
          }
        }
        n181 = flat-sequence {
          tunnel: w624 -> [w631]
          tunnel: [w633] -> w618
          tunnel: [w632] -> w623
          frame #0 {
            w630 = i16 0 items=["INTERNAL", "EXTERNAL", "HOLD/MANUAL"] ("trigger (internal:0)")
            w636 = i16 1 items=["DEG Q", "RAD D", "         R/G"] ("function B (deg q:0)")
            w637 = i16 3 items=["Z/Y", "R/G", "L", "C"] ("function A (z/y:0)")
            n182 = call "HP4192A Measure.vi"("OSC level (V)"=1.0, "test signal\nfreq (Hz)"="Freq Value (Hz) (10kHz)", "GPIB addess"=w631, "trigger (internal:0)"=w630, "function B (deg q:0)"=w636, "function A (z/y:0)"=w637) -> ("display B"=w633:dbl, "display A"=w632:dbl)  [unwired: 4 in]
            n183 = Wait (ms)(milliseconds to wait=u32 1000) -> ()  [unwired: 1 out]
          }
        }
        n184 = local read "Thickness"() -> (w629:dbl)
        n185 = local read "Area"() -> (w627:dbl)
        n186 = Multiply(x=w623, y=w629) -> (x*y=w628:dbl)
        n187 = Divide(x=w628, y=w627) -> (x/y=w626:dbl)
        n188 = Divide(x=w626, y=8.854e-12) -> (x/y=w619:dbl)
        "K10k" <- w619
        n189 = Wait (ms)(milliseconds to wait=u32 2000) -> ()  [unwired: 1 out]
        "C10k" <- w623
        "tand10k" <- w618
      }
      frame #9 {
        n190 = flat-sequence {
          tunnel: w667 -> [w687]
          tunnel: [w686] -> _
          tunnel: [w685] -> w665
          tunnel: w666 -> [w684]
          tunnel: [w684] -> w669
          frame #0 {
            n191 = call-poly "VISA Configure Serial Port"("VISA resource name"=w687, "data bits (8)"=7, "parity (0:none)"=1) -> ("error out"=w692:errorcluster)  [unwired: 11 in, 1 out]
            n192 = Concatenate Strings("*X01", "\r") -> (w695:string)
            n193 = VISA Write(VISA resource name=w687, write buffer=w695, error in (no error)=w692) -> (VISA resource name out=w706:refnum<visa-resource-name>, error out=w696:errorcluster)  [unwired: 1 out]
            n194 = property class="Instr"(reference=w706, error in=w696) -> (error out=w697:errorcluster, "Serial Settings:Number of Bytes at Serial Port"=w698:u32)  [unwired: 1 out]
            n195 = VISA Read(VISA resource name=w687, byte count=w698, error in (no error)=w697) -> (read buffer=w699:string, error out=w686:errorcluster)  [unwired: 2 out]
            n196 = String Length(string=w699) -> (length=w701:i32)
            n197 = Subtract(x=w701, y=4) -> (x-y=w703:i32)
            n198 = String Subset(string=w699, offset (0)=3, length (rest)=w703) -> (substring=w704:string)
            n199 = Concatenate Strings(w704, "\t") -> (w688:string)
            n200 = Scan Value(string=w688, format string="%f") -> (value=w685:dbl)  [unwired: 1 in, 1 out]
            "Temp25kHz" <- w685
          }
        }
        n201 = flat-sequence {
          tunnel: w669 -> [w676]
          tunnel: [w678] -> w663
          tunnel: [w677] -> w668
          frame #0 {
            w675 = i16 0 items=["INTERNAL", "EXTERNAL", "HOLD/MANUAL"] ("trigger (internal:0)")
            w681 = i16 1 items=["DEG Q", "RAD D", "         R/G"] ("function B (deg q:0)")
            w682 = i16 3 items=["Z/Y", "R/G", "L", "C"] ("function A (z/y:0)")
            n202 = call "HP4192A Measure.vi"("OSC level (V)"=1.0, "test signal\nfreq (Hz)"="Freq Value (Hz) (25kHz)", "GPIB addess"=w676, "trigger (internal:0)"=w675, "function B (deg q:0)"=w681, "function A (z/y:0)"=w682) -> ("display B"=w678:dbl, "display A"=w677:dbl)  [unwired: 4 in]
            n203 = Wait (ms)(milliseconds to wait=u32 1000) -> ()  [unwired: 1 out]
          }
        }
        n204 = local read "Thickness"() -> (w674:dbl)
        n205 = local read "Area"() -> (w672:dbl)
        n206 = Multiply(x=w668, y=w674) -> (x*y=w673:dbl)
        n207 = Divide(x=w673, y=w672) -> (x/y=w671:dbl)
        n208 = Divide(x=w671, y=8.854e-12) -> (x/y=w664:dbl)
        "K25k" <- w664
        n209 = Wait (ms)(milliseconds to wait=u32 2000) -> ()  [unwired: 1 out]
        "C25k" <- w668
        "tand25k" <- w663
      }
      frame #10 {
        n210 = flat-sequence {
          tunnel: w712 -> [w732]
          tunnel: [w731] -> _
          tunnel: [w730] -> w710
          tunnel: w711 -> [w729]
          tunnel: [w729] -> w714
          frame #0 {
            n211 = call-poly "VISA Configure Serial Port"("VISA resource name"=w732, "data bits (8)"=7, "parity (0:none)"=1) -> ("error out"=w737:errorcluster)  [unwired: 11 in, 1 out]
            n212 = Concatenate Strings("*X01", "\r") -> (w740:string)
            n213 = VISA Write(VISA resource name=w732, write buffer=w740, error in (no error)=w737) -> (VISA resource name out=w751:refnum<visa-resource-name>, error out=w741:errorcluster)  [unwired: 1 out]
            n214 = property class="Instr"(reference=w751, error in=w741) -> (error out=w742:errorcluster, "Serial Settings:Number of Bytes at Serial Port"=w743:u32)  [unwired: 1 out]
            n215 = VISA Read(VISA resource name=w732, byte count=w743, error in (no error)=w742) -> (read buffer=w744:string, error out=w731:errorcluster)  [unwired: 2 out]
            n216 = String Length(string=w744) -> (length=w746:i32)
            n217 = Subtract(x=w746, y=4) -> (x-y=w748:i32)
            n218 = String Subset(string=w744, offset (0)=3, length (rest)=w748) -> (substring=w749:string)
            n219 = Concatenate Strings(w749, "\t") -> (w733:string)
            n220 = Scan Value(string=w733, format string="%f") -> (value=w730:dbl)  [unwired: 1 in, 1 out]
            "Temp50kHz" <- w730
          }
        }
        n221 = flat-sequence {
          tunnel: w714 -> [w721]
          tunnel: [w724] -> w708
          tunnel: [w723] -> w713
          frame #0 {
            w720 = i16 0 items=["INTERNAL", "EXTERNAL", "HOLD/MANUAL"] ("trigger (internal:0)")
            w726 = i16 1 items=["DEG Q", "RAD D", "         R/G"] ("function B (deg q:0)")
            w727 = i16 3 items=["Z/Y", "R/G", "L", "C"] ("function A (z/y:0)")
            n222 = call "HP4192A Measure.vi"("OSC level (V)"=1.0, "test signal\nfreq (Hz)"="Freq Value (Hz) (50kHz)", "GPIB addess"=w721, "trigger (internal:0)"=w720, "function B (deg q:0)"=w726, "function A (z/y:0)"=w727) -> ("display B"=w724:dbl, "display A"=w723:dbl)  [unwired: 4 in]
            n223 = Wait (ms)(milliseconds to wait=u32 1000) -> ()  [unwired: 1 out]
          }
        }
        n224 = local read "Thickness"() -> (w719:dbl)
        n225 = local read "Area"() -> (w717:dbl)
        n226 = Multiply(x=w713, y=w719) -> (x*y=w718:dbl)
        n227 = Divide(x=w718, y=w717) -> (x/y=w716:dbl)
        n228 = Divide(x=w716, y=8.854e-12) -> (x/y=w709:dbl)
        "K50k" <- w709
        n229 = Wait (ms)(milliseconds to wait=u32 2000) -> ()  [unwired: 1 out]
        "C50k" <- w713
        "tand50k" <- w708
      }
      frame #11 {
        n230 = flat-sequence {
          tunnel: w757 -> [w777]
          tunnel: [w776] -> _
          tunnel: [w775] -> w755
          tunnel: w756 -> [w774]
          tunnel: [w774] -> w759
          frame #0 {
            n231 = call-poly "VISA Configure Serial Port"("VISA resource name"=w777, "data bits (8)"=7, "parity (0:none)"=1) -> ("error out"=w782:errorcluster)  [unwired: 11 in, 1 out]
            n232 = Concatenate Strings("*X01", "\r") -> (w785:string)
            n233 = VISA Write(VISA resource name=w777, write buffer=w785, error in (no error)=w782) -> (VISA resource name out=w796:refnum<visa-resource-name>, error out=w786:errorcluster)  [unwired: 1 out]
            n234 = property class="Instr"(reference=w796, error in=w786) -> (error out=w787:errorcluster, "Serial Settings:Number of Bytes at Serial Port"=w788:u32)  [unwired: 1 out]
            n235 = VISA Read(VISA resource name=w777, byte count=w788, error in (no error)=w787) -> (read buffer=w789:string, error out=w776:errorcluster)  [unwired: 2 out]
            n236 = String Length(string=w789) -> (length=w791:i32)
            n237 = Subtract(x=w791, y=4) -> (x-y=w793:i32)
            n238 = String Subset(string=w789, offset (0)=3, length (rest)=w793) -> (substring=w794:string)
            n239 = Concatenate Strings(w794, "\t") -> (w778:string)
            n240 = Scan Value(string=w778, format string="%f") -> (value=w775:dbl)  [unwired: 1 in, 1 out]
            "Temp100kHz" <- w775
          }
        }
        n241 = flat-sequence {
          tunnel: w759 -> [w766]
          tunnel: [w768] -> w753
          tunnel: [w767] -> w758
          frame #0 {
            w765 = i16 0 items=["INTERNAL", "EXTERNAL", "HOLD/MANUAL"] ("trigger (internal:0)")
            w771 = i16 1 items=["DEG Q", "RAD D", "         R/G"] ("function B (deg q:0)")
            w772 = i16 3 items=["Z/Y", "R/G", "L", "C"] ("function A (z/y:0)")
            n242 = call "HP4192A Measure.vi"("OSC level (V)"=1.0, "test signal\nfreq (Hz)"="Freq Value (Hz) (100kHz)", "GPIB addess"=w766, "trigger (internal:0)"=w765, "function B (deg q:0)"=w771, "function A (z/y:0)"=w772) -> ("display B"=w768:dbl, "display A"=w767:dbl)  [unwired: 4 in]
            n243 = Wait (ms)(milliseconds to wait=u32 1000) -> ()  [unwired: 1 out]
          }
        }
        n244 = local read "Thickness"() -> (w764:dbl)
        n245 = local read "Area"() -> (w762:dbl)
        n246 = Multiply(x=w758, y=w764) -> (x*y=w763:dbl)
        n247 = Divide(x=w763, y=w762) -> (x/y=w761:dbl)
        n248 = Divide(x=w761, y=8.854e-12) -> (x/y=w754:dbl)
        "K100k" <- w754
        n249 = Wait (ms)(milliseconds to wait=u32 2000) -> ()  [unwired: 1 out]
        "C100k" <- w758
        "tand100k" <- w753
      }
      frame #12 {
        n250 = flat-sequence {
          tunnel: w802 -> [w822]
          tunnel: [w821] -> _
          tunnel: [w820] -> w800
          tunnel: w801 -> [w819]
          tunnel: [w819] -> w804
          frame #0 {
            n251 = call-poly "VISA Configure Serial Port"("VISA resource name"=w822, "data bits (8)"=7, "parity (0:none)"=1) -> ("error out"=w827:errorcluster)  [unwired: 11 in, 1 out]
            n252 = Concatenate Strings("*X01", "\r") -> (w830:string)
            n253 = VISA Write(VISA resource name=w822, write buffer=w830, error in (no error)=w827) -> (VISA resource name out=w841:refnum<visa-resource-name>, error out=w831:errorcluster)  [unwired: 1 out]
            n254 = property class="Instr"(reference=w841, error in=w831) -> (error out=w832:errorcluster, "Serial Settings:Number of Bytes at Serial Port"=w833:u32)  [unwired: 1 out]
            n255 = VISA Read(VISA resource name=w822, byte count=w833, error in (no error)=w832) -> (read buffer=w834:string, error out=w821:errorcluster)  [unwired: 2 out]
            n256 = String Length(string=w834) -> (length=w836:i32)
            n257 = Subtract(x=w836, y=4) -> (x-y=w838:i32)
            n258 = String Subset(string=w834, offset (0)=3, length (rest)=w838) -> (substring=w839:string)
            n259 = Concatenate Strings(w839, "\t") -> (w823:string)
            n260 = Scan Value(string=w823, format string="%f") -> (value=w820:dbl)  [unwired: 1 in, 1 out]
            "Temp250kHz" <- w820
          }
        }
        n261 = flat-sequence {
          tunnel: w804 -> [w811]
          tunnel: [w814] -> w798
          tunnel: [w813] -> w803
          frame #0 {
            w810 = i16 0 items=["INTERNAL", "EXTERNAL", "HOLD/MANUAL"] ("trigger (internal:0)")
            w816 = i16 1 items=["DEG Q", "RAD D", "         R/G"] ("function B (deg q:0)")
            w817 = i16 3 items=["Z/Y", "R/G", "L", "C"] ("function A (z/y:0)")
            n262 = call "HP4192A Measure.vi"("OSC level (V)"=1.0, "test signal\nfreq (Hz)"="Freq Value (Hz) (250kHz)", "GPIB addess"=w811, "trigger (internal:0)"=w810, "function B (deg q:0)"=w816, "function A (z/y:0)"=w817) -> ("display B"=w814:dbl, "display A"=w813:dbl)  [unwired: 4 in]
            n263 = Wait (ms)(milliseconds to wait=u32 1000) -> ()  [unwired: 1 out]
          }
        }
        n264 = local read "Thickness"() -> (w809:dbl)
        n265 = local read "Area"() -> (w807:dbl)
        n266 = Multiply(x=w803, y=w809) -> (x*y=w808:dbl)
        n267 = Divide(x=w808, y=w807) -> (x/y=w806:dbl)
        n268 = Divide(x=w806, y=8.854e-12) -> (x/y=w799:dbl)
        "K250k" <- w799
        n269 = Wait (ms)(milliseconds to wait=u32 2000) -> ()  [unwired: 1 out]
        "C250k" <- w803
        "tand250k" <- w798
      }
      frame #13 {
        n270 = flat-sequence {
          tunnel: w847 -> [w867]
          tunnel: [w866] -> _
          tunnel: [w865] -> w845
          tunnel: w846 -> [w864]
          tunnel: [w864] -> w849
          frame #0 {
            n271 = call-poly "VISA Configure Serial Port"("VISA resource name"=w867, "data bits (8)"=7, "parity (0:none)"=1) -> ("error out"=w872:errorcluster)  [unwired: 11 in, 1 out]
            n272 = Concatenate Strings("*X01", "\r") -> (w875:string)
            n273 = VISA Write(VISA resource name=w867, write buffer=w875, error in (no error)=w872) -> (VISA resource name out=w886:refnum<visa-resource-name>, error out=w876:errorcluster)  [unwired: 1 out]
            n274 = property class="Instr"(reference=w886, error in=w876) -> (error out=w877:errorcluster, "Serial Settings:Number of Bytes at Serial Port"=w878:u32)  [unwired: 1 out]
            n275 = VISA Read(VISA resource name=w867, byte count=w878, error in (no error)=w877) -> (read buffer=w879:string, error out=w866:errorcluster)  [unwired: 2 out]
            n276 = String Length(string=w879) -> (length=w881:i32)
            n277 = Subtract(x=w881, y=4) -> (x-y=w883:i32)
            n278 = String Subset(string=w879, offset (0)=3, length (rest)=w883) -> (substring=w884:string)
            n279 = Concatenate Strings(w884, "\t") -> (w868:string)
            n280 = Scan Value(string=w868, format string="%f") -> (value=w865:dbl)  [unwired: 1 in, 1 out]
            "Temp500kHz" <- w865
          }
        }
        n281 = flat-sequence {
          tunnel: w849 -> [w856]
          tunnel: [w858] -> w843
          tunnel: [w857] -> w848
          frame #0 {
            w855 = i16 0 items=["INTERNAL", "EXTERNAL", "HOLD/MANUAL"] ("trigger (internal:0)")
            w861 = i16 1 items=["DEG Q", "RAD D", "         R/G"] ("function B (deg q:0)")
            w862 = i16 3 items=["Z/Y", "R/G", "L", "C"] ("function A (z/y:0)")
            n282 = call "HP4192A Measure.vi"("OSC level (V)"=1.0, "test signal\nfreq (Hz)"="Freq Value (Hz) (500kHz)", "GPIB addess"=w856, "trigger (internal:0)"=w855, "function B (deg q:0)"=w861, "function A (z/y:0)"=w862) -> ("display B"=w858:dbl, "display A"=w857:dbl)  [unwired: 4 in]
            n283 = Wait (ms)(milliseconds to wait=u32 1000) -> ()  [unwired: 1 out]
          }
        }
        n284 = local read "Thickness"() -> (w854:dbl)
        n285 = local read "Area"() -> (w852:dbl)
        n286 = Multiply(x=w848, y=w854) -> (x*y=w853:dbl)
        n287 = Divide(x=w853, y=w852) -> (x/y=w851:dbl)
        n288 = Divide(x=w851, y=8.854e-12) -> (x/y=w844:dbl)
        "K500k" <- w844
        n289 = Wait (ms)(milliseconds to wait=u32 2000) -> ()  [unwired: 1 out]
        "C500k" <- w848
        "tand500k" <- w843
      }
      frame #14 {
        n290 = flat-sequence {
          tunnel: w892 -> [w912]
          tunnel: [w911] -> _
          tunnel: [w910] -> w890
          tunnel: w891 -> [w909]
          tunnel: [w909] -> w894
          frame #0 {
            n291 = call-poly "VISA Configure Serial Port"("VISA resource name"=w912, "data bits (8)"=7, "parity (0:none)"=1) -> ("error out"=w917:errorcluster)  [unwired: 11 in, 1 out]
            n292 = Concatenate Strings("*X01", "\r") -> (w920:string)
            n293 = VISA Write(VISA resource name=w912, write buffer=w920, error in (no error)=w917) -> (VISA resource name out=w931:refnum<visa-resource-name>, error out=w921:errorcluster)  [unwired: 1 out]
            n294 = property class="Instr"(reference=w931, error in=w921) -> (error out=w922:errorcluster, "Serial Settings:Number of Bytes at Serial Port"=w923:u32)  [unwired: 1 out]
            n295 = VISA Read(VISA resource name=w912, byte count=w923, error in (no error)=w922) -> (read buffer=w924:string, error out=w911:errorcluster)  [unwired: 2 out]
            n296 = String Length(string=w924) -> (length=w926:i32)
            n297 = Subtract(x=w926, y=4) -> (x-y=w928:i32)
            n298 = String Subset(string=w924, offset (0)=3, length (rest)=w928) -> (substring=w929:string)
            n299 = Concatenate Strings(w929, "\t") -> (w913:string)
            n300 = Scan Value(string=w913, format string="%f") -> (value=w910:dbl)  [unwired: 1 in, 1 out]
            "Temp1MHz" <- w910
          }
        }
        n301 = flat-sequence {
          tunnel: w894 -> [w907]
          tunnel: [w901] -> w888
          tunnel: [w902] -> w893
          frame #0 {
            w900 = i16 0 items=["INTERNAL", "EXTERNAL", "HOLD/MANUAL"] ("trigger (internal:0)")
            w905 = i16 1 items=["DEG Q", "RAD D", "         R/G"] ("function B (deg q:0)")
            w906 = i16 3 items=["Z/Y", "R/G", "L", "C"] ("function A (z/y:0)")
            n302 = call "HP4192A Measure.vi"("OSC level (V)"=1.0, "test signal\nfreq (Hz)"="Freq Value (Hz) (1MHz)", "GPIB addess"=w907, "trigger (internal:0)"=w900, "function B (deg q:0)"=w905, "function A (z/y:0)"=w906) -> ("display B"=w901:dbl, "display A"=w902:dbl)  [unwired: 4 in]
            n303 = Wait (ms)(milliseconds to wait=u32 1000) -> ()  [unwired: 1 out]
          }
        }
        n304 = local read "Thickness"() -> (w899:dbl)
        n305 = local read "Area"() -> (w897:dbl)
        n306 = Multiply(x=w893, y=w899) -> (x*y=w898:dbl)
        n307 = Divide(x=w898, y=w897) -> (x/y=w896:dbl)
        n308 = Divide(x=w896, y=8.854e-12) -> (x/y=w889:dbl)
        "K1M" <- w889
        n309 = Wait (ms)(milliseconds to wait=u32 2000) -> ()  [unwired: 1 out]
        "C1M" <- w893
        "tand1M" <- w888
      }
    }
    n310 = flat-sequence {
      tunnel: w76 -> [w244]
      tunnel: w72 -> [w242]
      tunnel: w79 -> [w253]
      tunnel: w75 -> [w252]
      tunnel: w71 -> [w241]
      tunnel: w78 -> [w190]
      tunnel: w74 -> [w185]
      tunnel: w70 -> [w178]
      tunnel: w77 -> [w245]
      tunnel: w73 -> [w243]
      tunnel: w69 -> [w240]
      tunnel: w68 -> [w239]
      tunnel: w67 -> [w237]
      tunnel: w66 -> [w236]
      tunnel: w65 -> [w235]
      tunnel: w64 -> [w191]
      tunnel: w63 -> [w186]
      tunnel: w62 -> [w179]
      tunnel: w61 -> [w230]
      tunnel: w60 -> [w229]
      tunnel: w59 -> [w228]
      tunnel: w58 -> [w224]
      tunnel: w57 -> [w223]
      tunnel: w56 -> [w222]
      tunnel: w55 -> [w192]
      tunnel: w54 -> [w187]
      tunnel: w53 -> [w180]
      tunnel: w52 -> [w218]
      tunnel: w51 -> [w217]
      tunnel: w50 -> [w216]
      tunnel: w49 -> [w213]
      tunnel: w48 -> [w212]
      tunnel: w47 -> [w211]
      tunnel: w46 -> [w193]
      tunnel: w45 -> [w188]
      tunnel: w44 -> [w181]
      tunnel: w43 -> [w206]
      tunnel: w42 -> [w205]
      tunnel: w41 -> [w204]
      tunnel: w40 -> [w184]
      tunnel: w39 -> [w183]
      tunnel: w38 -> [w182]
      tunnel: w37 -> [w199]
      tunnel: w36 -> [w189]
      tunnel: w35 -> [w194]
      tunnel: [w184] -> w34
      tunnel: [w193] -> w33
      tunnel: [w192] -> w32
      tunnel: [w191] -> w31
      tunnel: [w190] -> w30
      tunnel: [w183] -> w29
      tunnel: [w188] -> w28
      tunnel: [w187] -> w27
      tunnel: [w186] -> w26
      tunnel: [w185] -> w25
      tunnel: [w182] -> w24
      tunnel: [w181] -> w23
      tunnel: [w180] -> w22
      tunnel: [w179] -> w21
      tunnel: [w178] -> w20
      frame #0 {
        w197 = 1000000000000.0 ("x")
        n311 = local read "C2.5k"() -> (w226:dbl)
        n312 = local read "C100k"() -> (w207:dbl)
        n313 = local read "C250k"() -> (w202:dbl)
        n314 = local read "C500k"() -> (w200:dbl)
        n315 = local read "C250"() -> (w233:dbl)
        n316 = local read "C10k"() -> (w219:dbl)
        n317 = local read "C25"() -> (w251:dbl)
        n318 = local read "C500"() -> (w238:dbl)
        n319 = local read "C25k"() -> (w214:dbl)
        n320 = local read "C100"() -> (w234:dbl)
        n321 = local read "C50k"() -> (w209:dbl)
        n322 = local read "C50"() -> (w246:dbl)
        n323 = local read "C1k"() -> (w231:dbl)
        n324 = local read "C5k"() -> (w221:dbl)
        n325 = local read "C1M"() -> (w196:dbl)
        n326 = Multiply(x=w197, y=w251) -> (x*y=w250:dbl)
        n327 = Multiply(x=w197, y=w246) -> (x*y=w249:dbl)
        n328 = Multiply(x=w197, y=w234) -> (x*y=w248:dbl)
        n329 = Multiply(x=w197, y=w238) -> (x*y=w232:dbl)
        n330 = Multiply(x=w197, y=w233) -> (x*y=w247:dbl)
        n331 = Multiply(x=w197, y=w231) -> (x*y=w227:dbl)
        n332 = Multiply(x=w197, y=w226) -> (x*y=w225:dbl)
        n333 = Multiply(x=w197, y=w221) -> (x*y=w220:dbl)
        n334 = Multiply(x=w197, y=w219) -> (x*y=w215:dbl)
        n335 = Multiply(x=w197, y=w214) -> (x*y=w210:dbl)
        n336 = Multiply(x=w197, y=w209) -> (x*y=w208:dbl)
        n337 = Multiply(x=w197, y=w207) -> (x*y=w203:dbl)
        n338 = Multiply(x=w197, y=w202) -> (x*y=w201:dbl)
        n339 = Multiply(x=w197, y=w200) -> (x*y=w198:dbl)
        n340 = Multiply(x=w197, y=w196) -> (x*y=w195:dbl)
        n341 = Build Array(w239, w250, w244, w242, w253, w249, w252, w241, w190, w248, w185, w178, w245, w247, w243, w240, w237, w232, w236, w235, w191, w227, w186, w179, w230, w225, w229, w228, w224, w220, w223, w222, w192, w215, w187, w180, w218, w210, w217, w216, w213, w208, w212, w211, w193, w203, w188, w181, w206, w201, w205, w204, w184, w198, w183, w182, w194, w195, w189, w199) -> (w256:dbl[])
        n342 = local read "Path & File Name (*.txt)"() -> (w254:path)
        n343 = call-poly <vilib>:"Write To Spreadsheet File.vi"("format (%.3f)"="%.10f", "append to file? (new file:F)"=TRUE, "1D data"=w256, "file path (dialog if empty)"=w254) -> ()  [unwired: 4 in, 1 out]
      }
    }
    n344 = flat-sequence {
      tunnel: w30 -> [w143]
      tunnel: w31 -> [w142]
      tunnel: w32 -> [w141]
      tunnel: w33 -> [w140]
      tunnel: w25 -> [w139]
      tunnel: w26 -> [w138]
      tunnel: w27 -> [w137]
      tunnel: w28 -> [w136]
      tunnel: w20 -> [w135]
      tunnel: w21 -> [w134]
      tunnel: w22 -> [w133]
      tunnel: w23 -> [w132]
      tunnel: w34 -> [w96]
      tunnel: w29 -> [w88]
      tunnel: w24 -> [w81]
      frame #0 {
        n345 = Insert Into Array(array="Temp10k", index=0, new element=w141) -> (w103:dbl[])
        n346 = Insert Into Array(array="Temp500k", index=0, new element=w96) -> (w93:dbl[])
        n347 = Insert Into Array(array="Temp100", index=0, new element=w143) -> (w105:dbl[])
        n348 = Insert Into Array(array="Temp1k", index=0, new element=w142) -> (w104:dbl[])
        n349 = Insert Into Array(array="Temp100k", index=0, new element=w140) -> (w102:dbl[])
        n350 = Insert Into Array(array="K100", index=0, new element=w139) -> (w125:dbl[])
        n351 = Insert Into Array(array="K10k", index=0, new element=w137) -> (w123:dbl[])
        n352 = Insert Into Array(array="K500k", index=0, new element=w88) -> (w87:dbl[])
        n353 = Insert Into Array(array="K1k", index=0, new element=w138) -> (w124:dbl[])
        n354 = Insert Into Array(array="K100k", index=0, new element=w136) -> (w122:dbl[])
        n355 = Build Array(w104) -> (w119:dbl[][])
        n356 = Build Array(w103) -> (w117:dbl[][])
        n357 = Build Array(w102) -> (w115:dbl[][])
        n358 = Build Array(w93) -> (w98:dbl[][])
        n359 = Build Array(w105) -> (w121:dbl[][])
        n360 = call "Convert to Dynamic Data19"("Array"=w87) -> ("Dynamic Data Type"=w91:dynamicdata)  [unwired: 3 in]
        n361 = Build Array(w104) -> (w108:dbl[][])
        n362 = Build Array(w103) -> (w110:dbl[][])
        n363 = Build Array(w102) -> (w112:dbl[][])
        n364 = Build Array(w93) -> (w92:dbl[][])
        n365 = call "Convert to Dynamic Data5"("Array"=w125) -> ("Dynamic Data Type"=w131:dynamicdata)  [unwired: 3 in]
        n366 = call "Convert to Dynamic Data6"("Array"=w124) -> ("Dynamic Data Type"=w130:dynamicdata)  [unwired: 3 in]
        n367 = call "Convert to Dynamic Data7"("Array"=w123) -> ("Dynamic Data Type"=w129:dynamicdata)  [unwired: 3 in]
        n368 = call "Convert to Dynamic Data8"("Array"=w122) -> ("Dynamic Data Type"=w128:dynamicdata)  [unwired: 3 in]
        n369 = Build Array(w105) -> (w106:dbl[][])
        n370 = Insert Into Array(array="tand100", index=0, new element=w135) -> (w161:dbl[])
        n371 = Insert Into Array(array="tand1k", index=0, new element=w134) -> (w162:dbl[])
        n372 = Insert Into Array(array="tand10k", index=0, new element=w133) -> (w163:dbl[])
        n373 = Insert Into Array(array="tand100k", index=0, new element=w132) -> (w164:dbl[])
        n374 = Insert Into Array(array="tand500k", index=0, new element=w81) -> (w82:dbl[])
        n375 = call "Convert to Dynamic Data9"("Array"=w161) -> ("Dynamic Data Type"=w146:dynamicdata)  [unwired: 3 in]
        n376 = call "Convert to Dynamic Data10"("Array"=w162) -> ("Dynamic Data Type"=w147:dynamicdata)  [unwired: 3 in]
        n377 = call "Convert to Dynamic Data11"("Array"=w163) -> ("Dynamic Data Type"=w100:dynamicdata)  [unwired: 3 in]
        n378 = call "Convert to Dynamic Data12"("Array"=w164) -> ("Dynamic Data Type"=w86:dynamicdata)  [unwired: 3 in]
        n379 = call "Convert to Dynamic Data20"("Array"=w82) -> ("Dynamic Data Type"=w85:dynamicdata)  [unwired: 3 in]
        n380 = call "Convert to Dynamic Data13"("2D Array"=w121) -> ("Dynamic Data Type"=w120:dynamicdata)  [unwired: 3 in]
        n381 = call "Convert to Dynamic Data"("2D Array"=w119) -> ("Dynamic Data Type"=w118:dynamicdata)  [unwired: 3 in]
        n382 = call "Convert to Dynamic Data2"("2D Array"=w117) -> ("Dynamic Data Type"=w116:dynamicdata)  [unwired: 3 in]
        n383 = call "Convert to Dynamic Data3"("2D Array"=w115) -> ("Dynamic Data Type"=w114:dynamicdata)  [unwired: 3 in]
        n384 = call "Convert to Dynamic Data17"("2D Array"=w98) -> ("Dynamic Data Type"=w99:dynamicdata)  [unwired: 3 in]
        n385 = call "Convert to Dynamic Data4"("2D Array"=w106) -> ("Dynamic Data Type"=w107:dynamicdata)  [unwired: 3 in]
        n386 = call "Convert to Dynamic Data14"("2D Array"=w108) -> ("Dynamic Data Type"=w109:dynamicdata)  [unwired: 3 in]
        n387 = call "Convert to Dynamic Data15"("2D Array"=w110) -> ("Dynamic Data Type"=w111:dynamicdata)  [unwired: 3 in]
        n388 = call "Convert to Dynamic Data16"("2D Array"=w112) -> ("Dynamic Data Type"=w113:dynamicdata)  [unwired: 3 in]
        n389 = call "Convert to Dynamic Data18"("2D Array"=w92) -> ("Dynamic Data Type"=w94:dynamicdata)  [unwired: 3 in]
        n390 = Merge Signals(w120, w118, w116, w114, w99) -> (w126:dynamicdata)
        n391 = Merge Signals(w131, w130, w129, w128, w91) -> (w127:dynamicdata)
        n392 = Merge Signals(w107, w109, w111, w113, w94) -> (w101:dynamicdata)
        n393 = Merge Signals(w146, w147, w100, w86, w85) -> (w148:dynamicdata)
        n394 = call "Build XY Graph"("Y Input"=w127, "X Input"=w126) -> ("XY Graph"=→"Relative Permittivity vs. Temperature":cluster{"Y":dbl[], "Y":dbl[]}[])  [unwired: 8 in, 1 out]
        n395 = call "Build XY Graph2"("Y Input"=w148, "X Input"=w101) -> ("XY Graph"=→"Dielectric Loss vs. Temperature":cluster{"Y":dbl[], "Y":dbl[]}[])  [unwired: 8 in, 1 out]
      }
    }
  }
  n396 = flat-sequence {
    tunnel: w2 -> [w993]
    tunnel: [w991] -> w1
    frame #0 {
      w960 = "\t"
      w961 = "Temperature (C)" ("string")
      n397 = local read "Thickness"() -> (w997:dbl)
      n398 = local read "Area"() -> (w998:dbl)
      n399 = Number To Exponential String(number=w998) -> (E-format string=w990:string)  [unwired: 3 in]
      n400 = Number To Exponential String(number=w997) -> (E-format string=w988:string)  [unwired: 3 in]
      n401 = Concatenate Strings("Thickness (m)" ("string"), "\t", w988) -> (w986:string)
      n402 = Concatenate Strings("Area (m^2)" ("string"), "\t", w990) -> (w994:string)
      n403 = Concatenate Strings("Comment" ("string"), "\t", "Comment (Sample's Name, compositions, whatever you want,..)", "\r", w994, "\t", w986, "\r", w961, w960, "C25Hz (pF)" ("string"), w960, "K25Hz" ("string"), w960, "tand25Hz" ("string"), w960, w961, w960, "C50Hz (pF)" ("string"), w960, "K50Hz" ("string"), w960, "tand50Hz" ("string"), w960, w961, w960, "C100Hz (pF)" ("string"), w960, "K100Hz" ("string"), w960, "tand100Hz" ("string"), w960, w961, w960, "C250Hz (pF)" ("string"), w960, "K250Hz" ("string"), w960, "tand250Hz" ("string"), w960, w961, w960, "C500Hz (pF)" ("string"), w960, "K500Hz" ("string"), w960, "tand500Hz" ("string"), w960, w961, w960, "C1kHz (pF)" ("string"), w960, "K1kHz" ("string"), w960, "tand1kHz" ("string"), w960, w961, w960, "C2.5kHz (pF)" ("string"), w960, "K2.5kHz" ("string"), w960, "tand2.5kHz" ("string"), w960, w961, w960, "C5kHz (pF)" ("string"), w960, "K5kHz" ("string"), w960, "tand5kHz" ("string"), w960, w961, w960, "C10kHz (pF)" ("string"), w960, "K10kHz" ("string"), w960, "tand10kHz" ("string"), w960, w961, w960, "C25kHz (pF)" ("string"), w960, "K25kHz" ("string"), w960, "tand25kHz" ("string"), w960, w961, w960, "C50kHz (pF)" ("string"), w960, "K50kHz" ("string"), w960, "tand50kHz" ("string"), w960, w961, w960, "C100kHz (pF)" ("string"), w960, "K100kHz" ("string"), w960, "tand100kHz" ("string"), w960, w961, w960, "C250kHz (pF)" ("string"), w960, "K250kHz" ("string"), w960, "tand250kHz" ("string"), w960, w961, w960, "C500kHz (pF)" ("string"), w960, "K500kHz" ("string"), w960, "tand500kHz" ("string"), w960, w961, w960, "C1MHz (pF)" ("string"), w960, "K1MHz" ("string"), w960, "tand1MHz" ("string"), "\r\n") -> (w992:string)
      n404 = Write to Text File(file (use dialog)=w993, text=w992) -> (error out=w991:errorcluster)  [unwired: 2 in, 2 out]
    }
  }
